vi "Controller_version1.vi"() -> ()   [LabVIEW 2020]
uses:
  <vilib>/Platform/TimedLoop/XDataNode/wakeup.ctl
  <vilib>/Platform/TimedLoop/XDataNode/XDNodeRunTimeDep.lvlib
  <vilib>/Platform/TimedLoop/XDataNode/nitl_modes.ctl
  <vilib>/Platform/TimedLoop/XDataNode/timing_clust.ctl
  <vilib>/Platform/TimedLoop/XDataNode/XDataNode.xnode
  <vilib>/addons/control/pid/NI_PID_pid.lvlib
  <vilib>/addons/control/pid/pid.llb/PID (DBL).vi
  <vilib>/imathl/engines/lvmath/Functions/Error Handling/Create Error.vi
  <vilib>/imath/engines/lvmath2/RunTimeEngine/BuiltInFunctions/diag/NIMS_diag.vi
  <vilib>/imath/engines/lvmath2/RunTimeEngine/NodeEndStatement/NIMS_NodeEndStatement_Output.vi
  <vilib>/imath/engines/lvmath2/RunTimeEngine/ErrorHandling/NIMS_Finalize Error.vi
  <vilib>/imath/engines/lvmath2/RunTimeEngine/IndexReplace/NIMS M($,S)=V.vi
  <vilib>/imath/engines/lvmath2/RunTimeEngine/IndexRead/NIMS V(S).vi
  <vilib>/imath/engines/lvmath2/RunTimeEngine/ErrorHandling/NIMS_Create Error From Enums.vi
  <vilib>/imath/engines/lvmath2/RunTimeEngine/RangeToken/NIMS_Range_R2 - Integer.vi
  <vilib>/imath/engines/lvmath2/RunTimeEngine/VariableToken/NIMS_VariableToken_CondDefinedDefinedByReplace.vi
  <vilib>/imath/engines/lvmath2/RunTimeEngine/IndexReplace/NIMS V(S)=S.vi
  <vilib>/imath/engines/lvmath2/RunTimeEngine/CommandStatement/MC_CommandStatement_break.vi
  <vilib>/imath/engines/lvmath2/RunTimeEngine/VariableToken/NIMS_VariableToken_CondDefined.vi
  <vilib>/imath/engines/lvmath2/RunTimeEngine/IndexRead/NIMS V($).vi
  <vilib>/imath/engines/lvmath2/RunTimeEngine/ArithmeticOperatorToken/NIMS_ArithmeticOperator_rightdiv(C,C).vi
  <vilib>/imath/engines/lvmath2/RunTimeEngine/ArithmeticOperatorToken/NIMS_ArithmeticOperator_minus.vi
  <vilib>/imath/engines/lvmath2/RunTimeEngine/ArithmeticOperatorToken/NIMS_ArithmeticOperator_times.vi
  <vilib>/imath/engines/lvmath2/RunTimeEngine/ArithmeticOperatorToken/NIMS_ArithmeticOperator_plus.vi
  <vilib>/imath/engines/lvmath2/RunTimeEngine/ArithmeticOperatorToken/NIMS_ArithmeticOperator_multmx(M,CV).vi
  <vilib>/imath/engines/lvmath2/RunTimeEngine/ArithmeticOperatorToken/NIMS_ArithmeticOperator_multmx(M,CV)-internal.vi
  <vilib>/imath/engines/lvmath2/RunTimeEngine/ArithmeticOperatorToken/NIMS_ArithmeticOperator_multmx.vi
  <vilib>/imath/engines/lvmath2/RunTimeEngine/ArithmeticOperatorToken/NIMS_ArithmeticOperator_rightdiv.vi
  <vilib>/imath/engines/lvmath2/RunTimeEngine/MatrixToken/NIMS_MatrixToken_SorCV_M.vi
  <vilib>/imath/engines/lvmath2/RunTimeEngine/IndexRead/NIMS V(R2).vi
  <vilib>/imath/engines/lvmath2/RunTimeEngine/BuiltInFunctions/reshapemx/NIMS_[GM]_reshapemx.vi
  <vilib>/imath/engines/lvmath2/RunTimeEngine/IndexRead/NIMS M(S,$).vi
  <vilib>/imath/engines/lvmath2/RunTimeEngine/ArithmeticOperatorToken/NIMS_ArithmeticOperator_multmx(RV,CV).vi
  <vilib>/imath/engines/lvmath2/RunTimeEngine/IndexReplace/NIMS V(S)=M.vi
  <vilib>/imath/engines/lvmath2/RunTimeEngine/IndexRead/NIMS M(S).vi
  <vilib>/imath/engines/lvmath2/RunTimeEngine/ArithmeticOperatorToken/NIMS_ArithmeticOperator_rightdivmx(C,C).vi
  <vilib>/imath/engines/lvmath2/RunTimeEngine/BuiltInFunctions/max/2 inputs/NIMS_max(CG,CG)-no size check.vi
  <vilib>/imath/engines/lvmath2/RunTimeEngine/BuiltInFunctions/min/2 inputs/NIMS_min(CG,CG)-no size check.vi
  <vilib>/imath/engines/lvmath2/RunTimeEngine/IndexReplace/NIMS M(S)=S.vi
  <vilib>/imath/engines/lvmath2/RunTimeEngine/NodeEndStatement/NIMS_NodeEndStatement_Get Vector.vi
  <vilib>/imath/engines/lvmath2/RunTimeEngine/NodeEndStatement/NIMS_NodeEndStatement_Get Scalar.vi
  <vilib>/imath/engines/lvmath/Functions/Error Handling/MergeErrorsWrapper.vi
panel:
  out "No error 3":bool
  out "No error 2":bool
  in  "Use\nPreset_Theta":bool
  out "Theta_Boom_F_hat_next":T1(graph)
  out "Theta_Boom_Q_hat_next":T1(graph)
  out "Theta_Stick_Q_hat_next":T1(graph)
  out "Theta_Stick_F_hat_next":T1(graph)
  out "e2_e3":dbl[](array[numeric])
  out "e3":dbl[](array[numeric])
  out "e2":dbl[](array[numeric])
  out "F_Boom":cluster{dbl, dbl, dbl, dbl}(graph)
  out "Q_Swing":cluster{dbl, dbl, dbl, dbl}(graph)
  in  "保存路径":path=path "C:/Qmz/data1.bin"
  in  "Save Data":bool
  in  "Stop\nTheta_Update":bool=TRUE
  out "Q_Boom":cluster{dbl, dbl, dbl, dbl}(graph)
  out "F_Stick":cluster{dbl, dbl, dbl, dbl}(graph)
  out "Q_Stick":cluster{dbl, dbl, dbl, dbl}(graph)
  out "F_Swing":cluster{dbl, dbl, dbl, dbl}(graph)
  out "Esti_e2":T2(graph)={"FLda1[0]"=125.504748463915, "FLda1[1]"=53.955555282260676, "FLda1[2]"=-93.06627669799211}
  out "Esti_e1":T2(graph)={"FLda1[0]"=125.504748463915, "FLda1[1]"=53.955555282260676, "FLda1[2]"=-93.06627669799211}
  out "Swing":T3(graph)
  out "Stick":T3(graph)
  out "Boom":T3(graph)
  in  "sw_Y_Q":bool
  in  "w2":dbl[](array[numeric])=[1414.0, 4000.0, 3020.0]
  in  "w1":dbl[](array[numeric])=[0.26, 1.1, 0.07]
  out "Theta_Boom_Q_hat_next":dbl[](array[numeric])
  out "Theta_Boom_F_hat_next":dbl[](array[numeric])
  out "Theta_Swing_Q_hat_next":dbl[](array[numeric])
  out "Theta_Swing_F_hat_next":dbl[](array[numeric])
  out "Theta_Stick_Q_hat_next":dbl[](array[numeric])
  out "Theta_Stick_F_hat_next":dbl[](array[numeric])
  out "ARC_U":dbl[](array[numeric])
  in  "sw_d2hat":bool
  in  "sw_d1hat":bool
  in  "gamma_d2(E-8)":dbl[](array[numeric])=[6.5, 3.1, 5.0]
  in  "gamma_d1":dbl[](array[numeric])=[250.0, 6000.1, 6000.1]
  in  "Theta_s2_init(E-8)":dbl[](array[numeric])=[2.0, 2.3, 2.5, 0.0, 100.0, 10.0, 0.0, -99.0, -200.0]
  in  "Theta_s1_init":dbl[](array[numeric])=[500.0, 66.0, 30.0, 53.0, 57.0, 31.0, -10.0, -73.0, 77.0]
  in  "sw_FLda1":bool=TRUE
  in  "sw_QLda1":bool=TRUE
  in  "STOP/Return to save position":bool=TRUE
  in  "Swing？(F)":bool=TRUE
  in  "Boom？(F)":bool
  in  "Stickj？(F)":bool=TRUE
  in  "K3(E-8)":dbl[](array[numeric])=[0.8, 1.0, 4.0] format="%#_8g"
  in  "K2":dbl[](array[numeric])=[650.0, 850.0, 800.0]
  in  "K1":dbl[](array[numeric])=[80.0, 80.0, 80.0]
  out "?":string="Now OpenLoop is running"
  out "?":string="Now OpenLoop is running"
  out "?":string="Now OpenLoop is running"
  in  "CloseLoop":T4 caption="ARC开关"
  out "Angle_Stick":dbl
  out "Angle_Boom":dbl
  out "Angle_Swing":dbl
  out "millisecond timer value":u32
  out "real time(s)":dbl
  out "minus":dbl format="%#_10g"
  out "No error":bool
  in  "PID gains":T5={"proportional gain (Kc)"=0.15, "integral time (Ti, min)"=0.003, "derivative time (Td, min)"=0.0005} caption="未越界" {"derivative time (Td, min)" format="%.6f"; "integral time (Ti, min)" format="%.6f"; "proportional gain (Kc)" step=0.01 format="%.6f"}
  out "?":bool
  in  "PID gains 2":T5={"proportional gain (Kc)"=0.16, "integral time (Ti, min)"=0.006, "derivative time (Td, min)"=0.0001} caption="未越界" {"derivative time (Td, min)" format="%.6f"; "integral time (Ti, min)" format="%.6f"; "proportional gain (Kc)" format="%.6f"}
  in  "PID gains 3":T5={"proportional gain (Kc)"=0.15, "integral time (Ti, min)"=0.003, "derivative time (Td, min)"=1e-05} caption="未越界" {"derivative time (Td, min)" step=0.001 format="%.6f"; "integral time (Ti, min)" step=0.001 format="%.6f"; "proportional gain (Kc)" step=0.01 format="%.6f"}
  out "?":bool
  out "?":bool
  in  "OpenLoop":T6={"Swing"=TRUE, "Boom"=TRUE, "Stick"=TRUE, "Swing_U"=-1.0, "Boom_U"=1.0, "Stick_U"=-1.0}
  in  "bias Swing":dbl
  in  "bias Boom":dbl
  in  "bias Stick":dbl
  in  "t-whole_Swing":i32=300
  in  "p_end Swing":dbl=-40.0
  in  "a_max Swing":dbl=-20.0
  in  "v_max Swing":dbl=-20.0
  in  "t-whole_Boom":i32=300
  in  "p_end Boom":dbl=-40.0
  in  "a_max Boom":dbl=-20.0
  in  "v_max Boom":dbl=-20.0
  in  "t-whole_Stick":i32=300
  in  "p_end_Stick":dbl=-40.0
  in  "a_max_Stick":dbl=-20.0
  in  "v_max_Stick":dbl=-20.0
  in  "pin1":dbl(slide)=40.50458715596331 scale=-60.0..55.0
  in  "Stick":T7={"Open P2P Traj"=TRUE, "Open Sine Traj"=FALSE, "Open Ramp Traj"=FALSE, "Open DIY Traj"=FALSE}
  in  "Boom":T7={"Open P2P Traj"=TRUE, "Open Sine Traj"=FALSE, "Open Ramp Traj"=FALSE, "Open DIY Traj"=FALSE}
  in  "Swing":T7={"Open P2P Traj"=TRUE, "Open Sine Traj"=FALSE, "Open Ramp Traj"=FALSE, "Open DIY Traj"=FALSE}
  in  "pin2":dbl(slide)=33.853211009174316 scale=-20.0..90.0
  in  "pin3":dbl(slide)=-87.9816513761468 scale=-160.0..-53.0
  # "s1 上到下\nfv\nfc\nD_n\ns2 上到下\n1/beta\nD_Q1\nD_Q2"
  # "上到下\n*Ld \\ *Lda1 \\ *Lds2 \\ *Lda2"
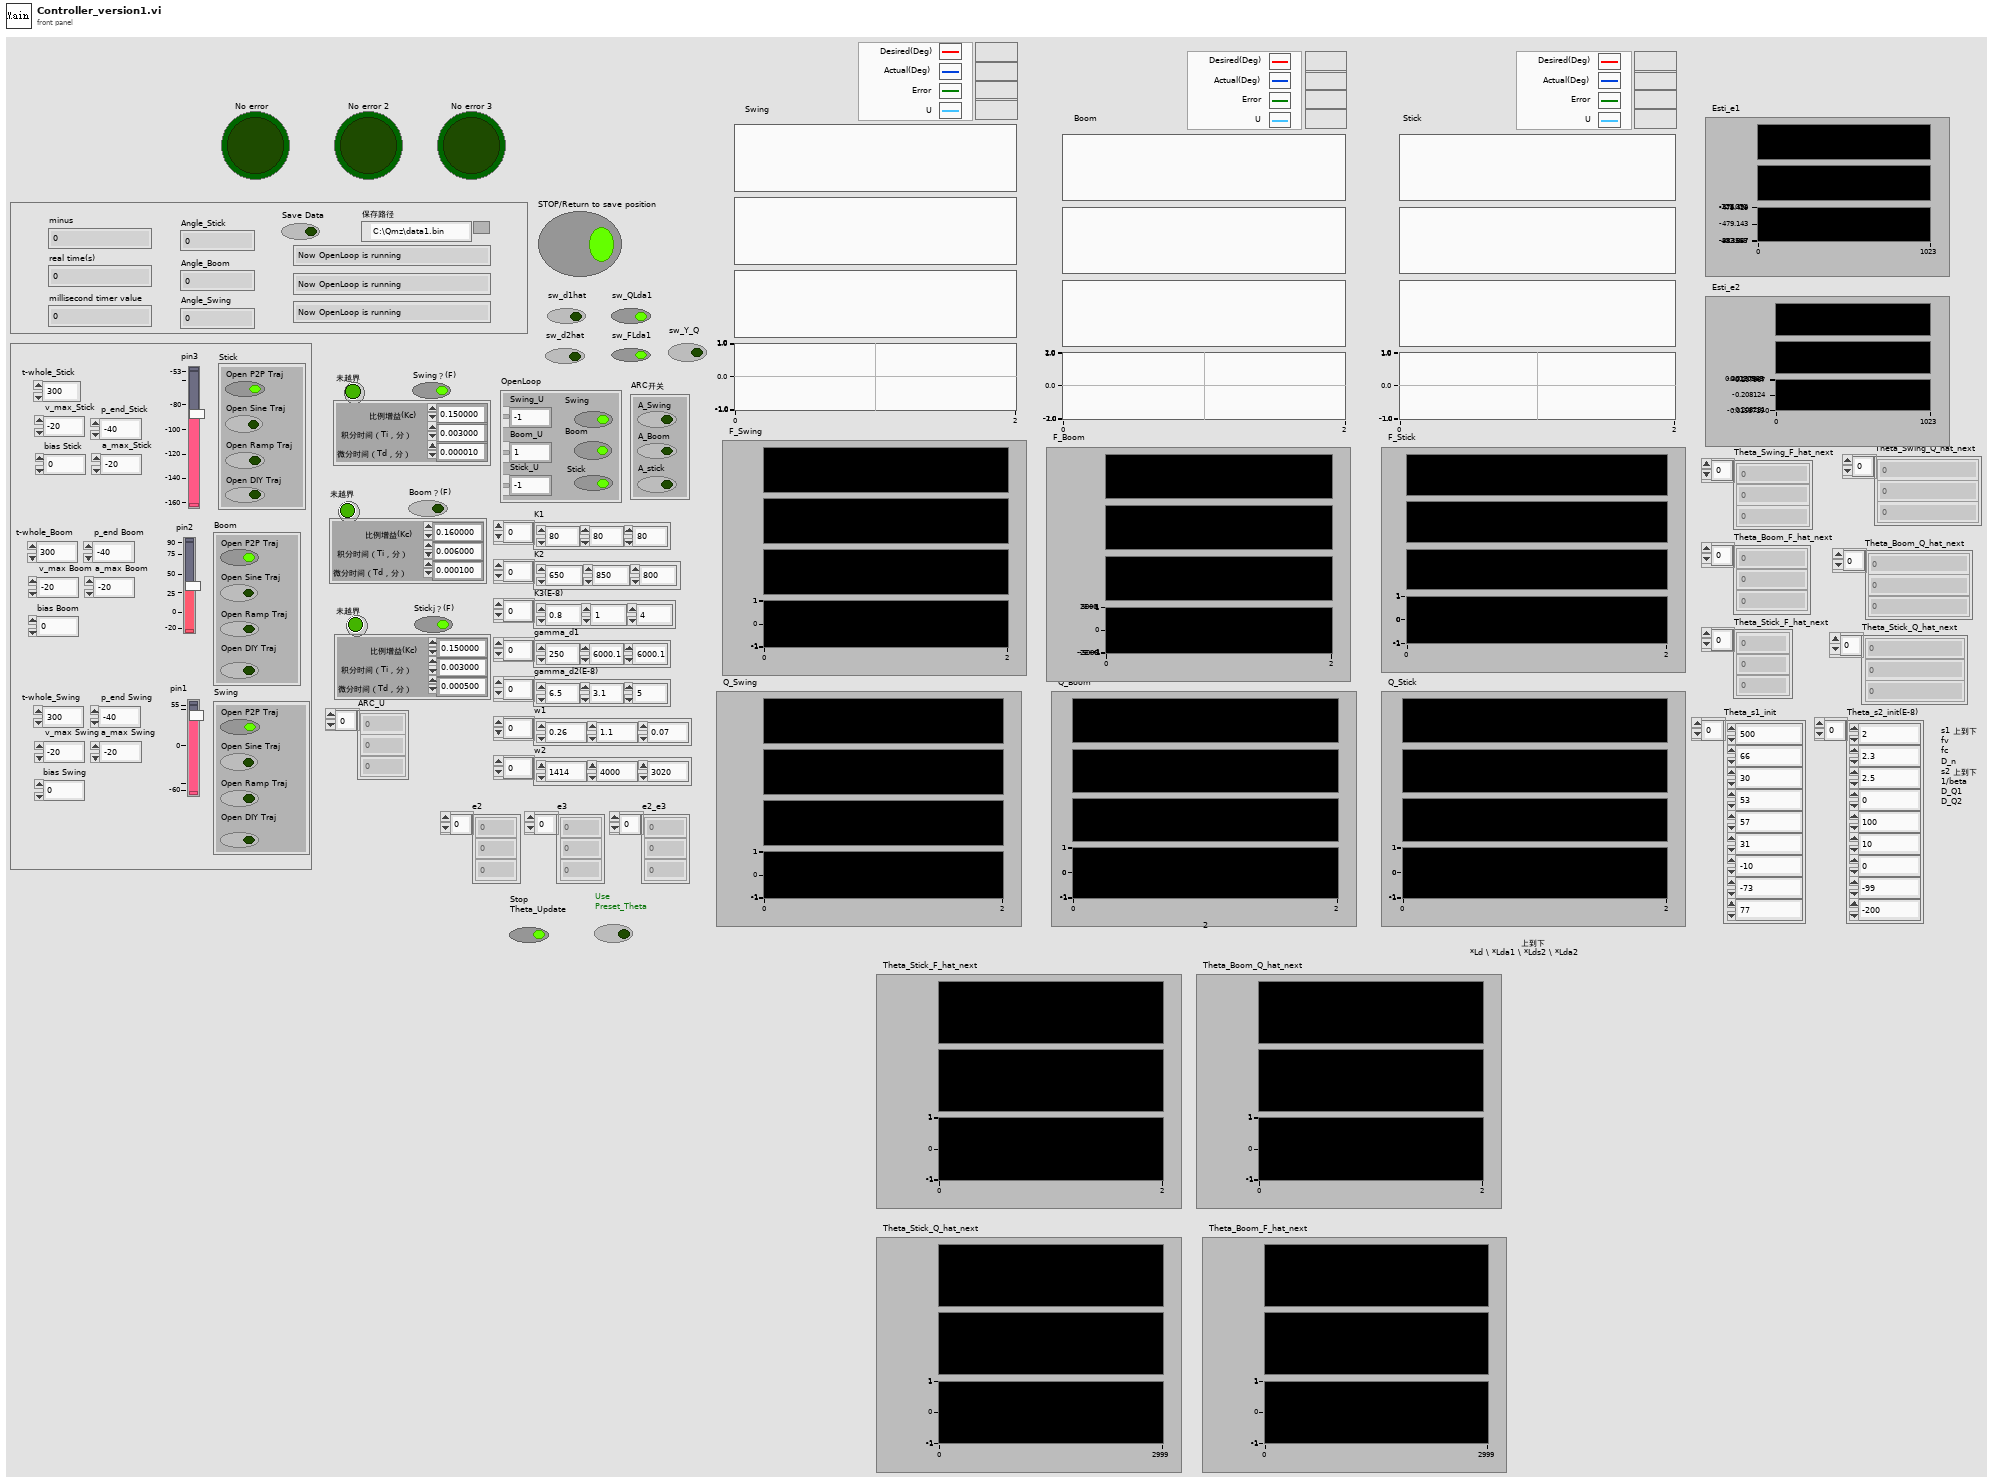
[diagram p1: front panel]
types:
  T1 = cluster{"Theta_Stick_F_hat_next[0]":dbl, "Theta_Stick_F_hat_next[1]":dbl, "Theta_Stick_F_hat_next[2]":dbl}
  T2 = cluster{"FLda1[0]":dbl, "FLda1[1]":dbl, "FLda1[2]":dbl}
  T3 = cluster{"Double":dbl, "Double":dbl, "Double":dbl, "Double":dbl}
  T4 = cluster{"A_Swing":bool, "A_Boom":bool, "A_stick\n":bool}
  T5 = cluster{"proportional gain (Kc)":dbl, "integral time (Ti, min)":dbl, "derivative time (Td, min)":dbl}
  T6 = cluster{"Swing":bool, "Boom":bool, "Stick":bool, "Swing_U":dbl, "Boom_U":dbl, "Stick_U":dbl}
  T7 = cluster{"Open P2P Traj":bool, "Open Sine Traj":bool, "Open Ramp Traj":bool, "Open DIY Traj":bool}
  T8 = typedef "XDNodeRunTimeDep.lvlib/timing_clust.ctl" = cluster{"Expected End [f-1]":u64, "Actual End [f-1]":u64, "Finished Late? [f-1]":bool, "Expected End [i-1]":u64, "Actual End [i-1]":u64, "Finished Late? [i-1]":bool, "Expected Start [i]":u64, "Actual Start [i]":u64, "Expected Start [f]":u64, "Actual Start [f]":u64, "Source Name":string, "Structure Name":string, "Period":i64, "Deadline":i64, "Offset":i64, "Start":i64, "Priority":i32, "Timeout":i32, "Mode":T9, "Wakeup Reason":T10, "Error":errorcluster, "Source Type":string, "Secondary Source Type":string, "Global End Time":u64, "Global Start Time":u64, "Frame Duration":u64, "Iteration Duration":u64, "Assigned CPU":i32, "I/O Scan Engine Mode":u32}
  T9 = typedef "XDNodeRunTimeDep.lvlib/nitl_modes.ctl" = enum32{"No Change", "Process missed periods, maintain original phase", "Discard missed periods, maintain original phase", "Process missed periods, ignore original phase", "Discard missed periods, ignore original phase"}
  T10 = typedef "XDNodeRunTimeDep.lvlib/wakeup.ctl" = enum32{"Normal", "Aborted", "Asynchronous wakeup", "Timing source error", "Timed loop error", "Timeout"}
  T11 = cluster{"Q_Stick[0]":cdb, "Q_Stick[1]":cdb, "Q_Stick[2]":cdb, "Q_Stick[3]":cdb}
  T12 = cluster{"Q_Boom[0]":cdb, "Q_Boom[1]":cdb, "Q_Boom[2]":cdb, "Q_Boom[3]":cdb}
  T13 = cluster{"Q_Swing[0]":cdb, "Q_Swing[1]":cdb, "Q_Swing[2]":cdb, "Q_Swing[3]":cdb}
  T14 = cluster{"F_Stick[0]":cdb, "F_Stick[1]":cdb, "F_Stick[2]":cdb, "F_Stick[3]":cdb}
  T15 = cluster{"F_Boom[0]":cdb, "F_Boom[1]":cdb, "F_Boom[2]":cdb, "F_Boom[3]":cdb}
  T16 = cluster{"F_Swing[0]":cdb, "F_Swing[1]":cdb, "F_Swing[2]":cdb, "F_Swing[3]":cdb}
  T17 = cluster{"Epsilon_1[0]":cdb, "Epsilon_1[1]":cdb, "Epsilon_1[2]":cdb}
  T18 = cluster{"Epsilon_2[0]":cdb, "Epsilon_2[1]":cdb, "Epsilon_2[2]":cdb}
  T19 = cluster{"Theta_Stick_Q_hat_next[0]":dbl, "Theta_Stick_Q_hat_next[1]":dbl, "Theta_Stick_Q_hat_next[2]":dbl}
  T20 = cluster{"Theta_Boom_Q_hat_next[0]":dbl, "Theta_Boom_Q_hat_next[1]":dbl, "Theta_Boom_Q_hat_next[2]":dbl}
  T21 = cluster{"Theta_Boom_F_hat_next[0]":dbl, "Theta_Boom_F_hat_next[1]":dbl, "Theta_Boom_F_hat_next[2]":dbl}
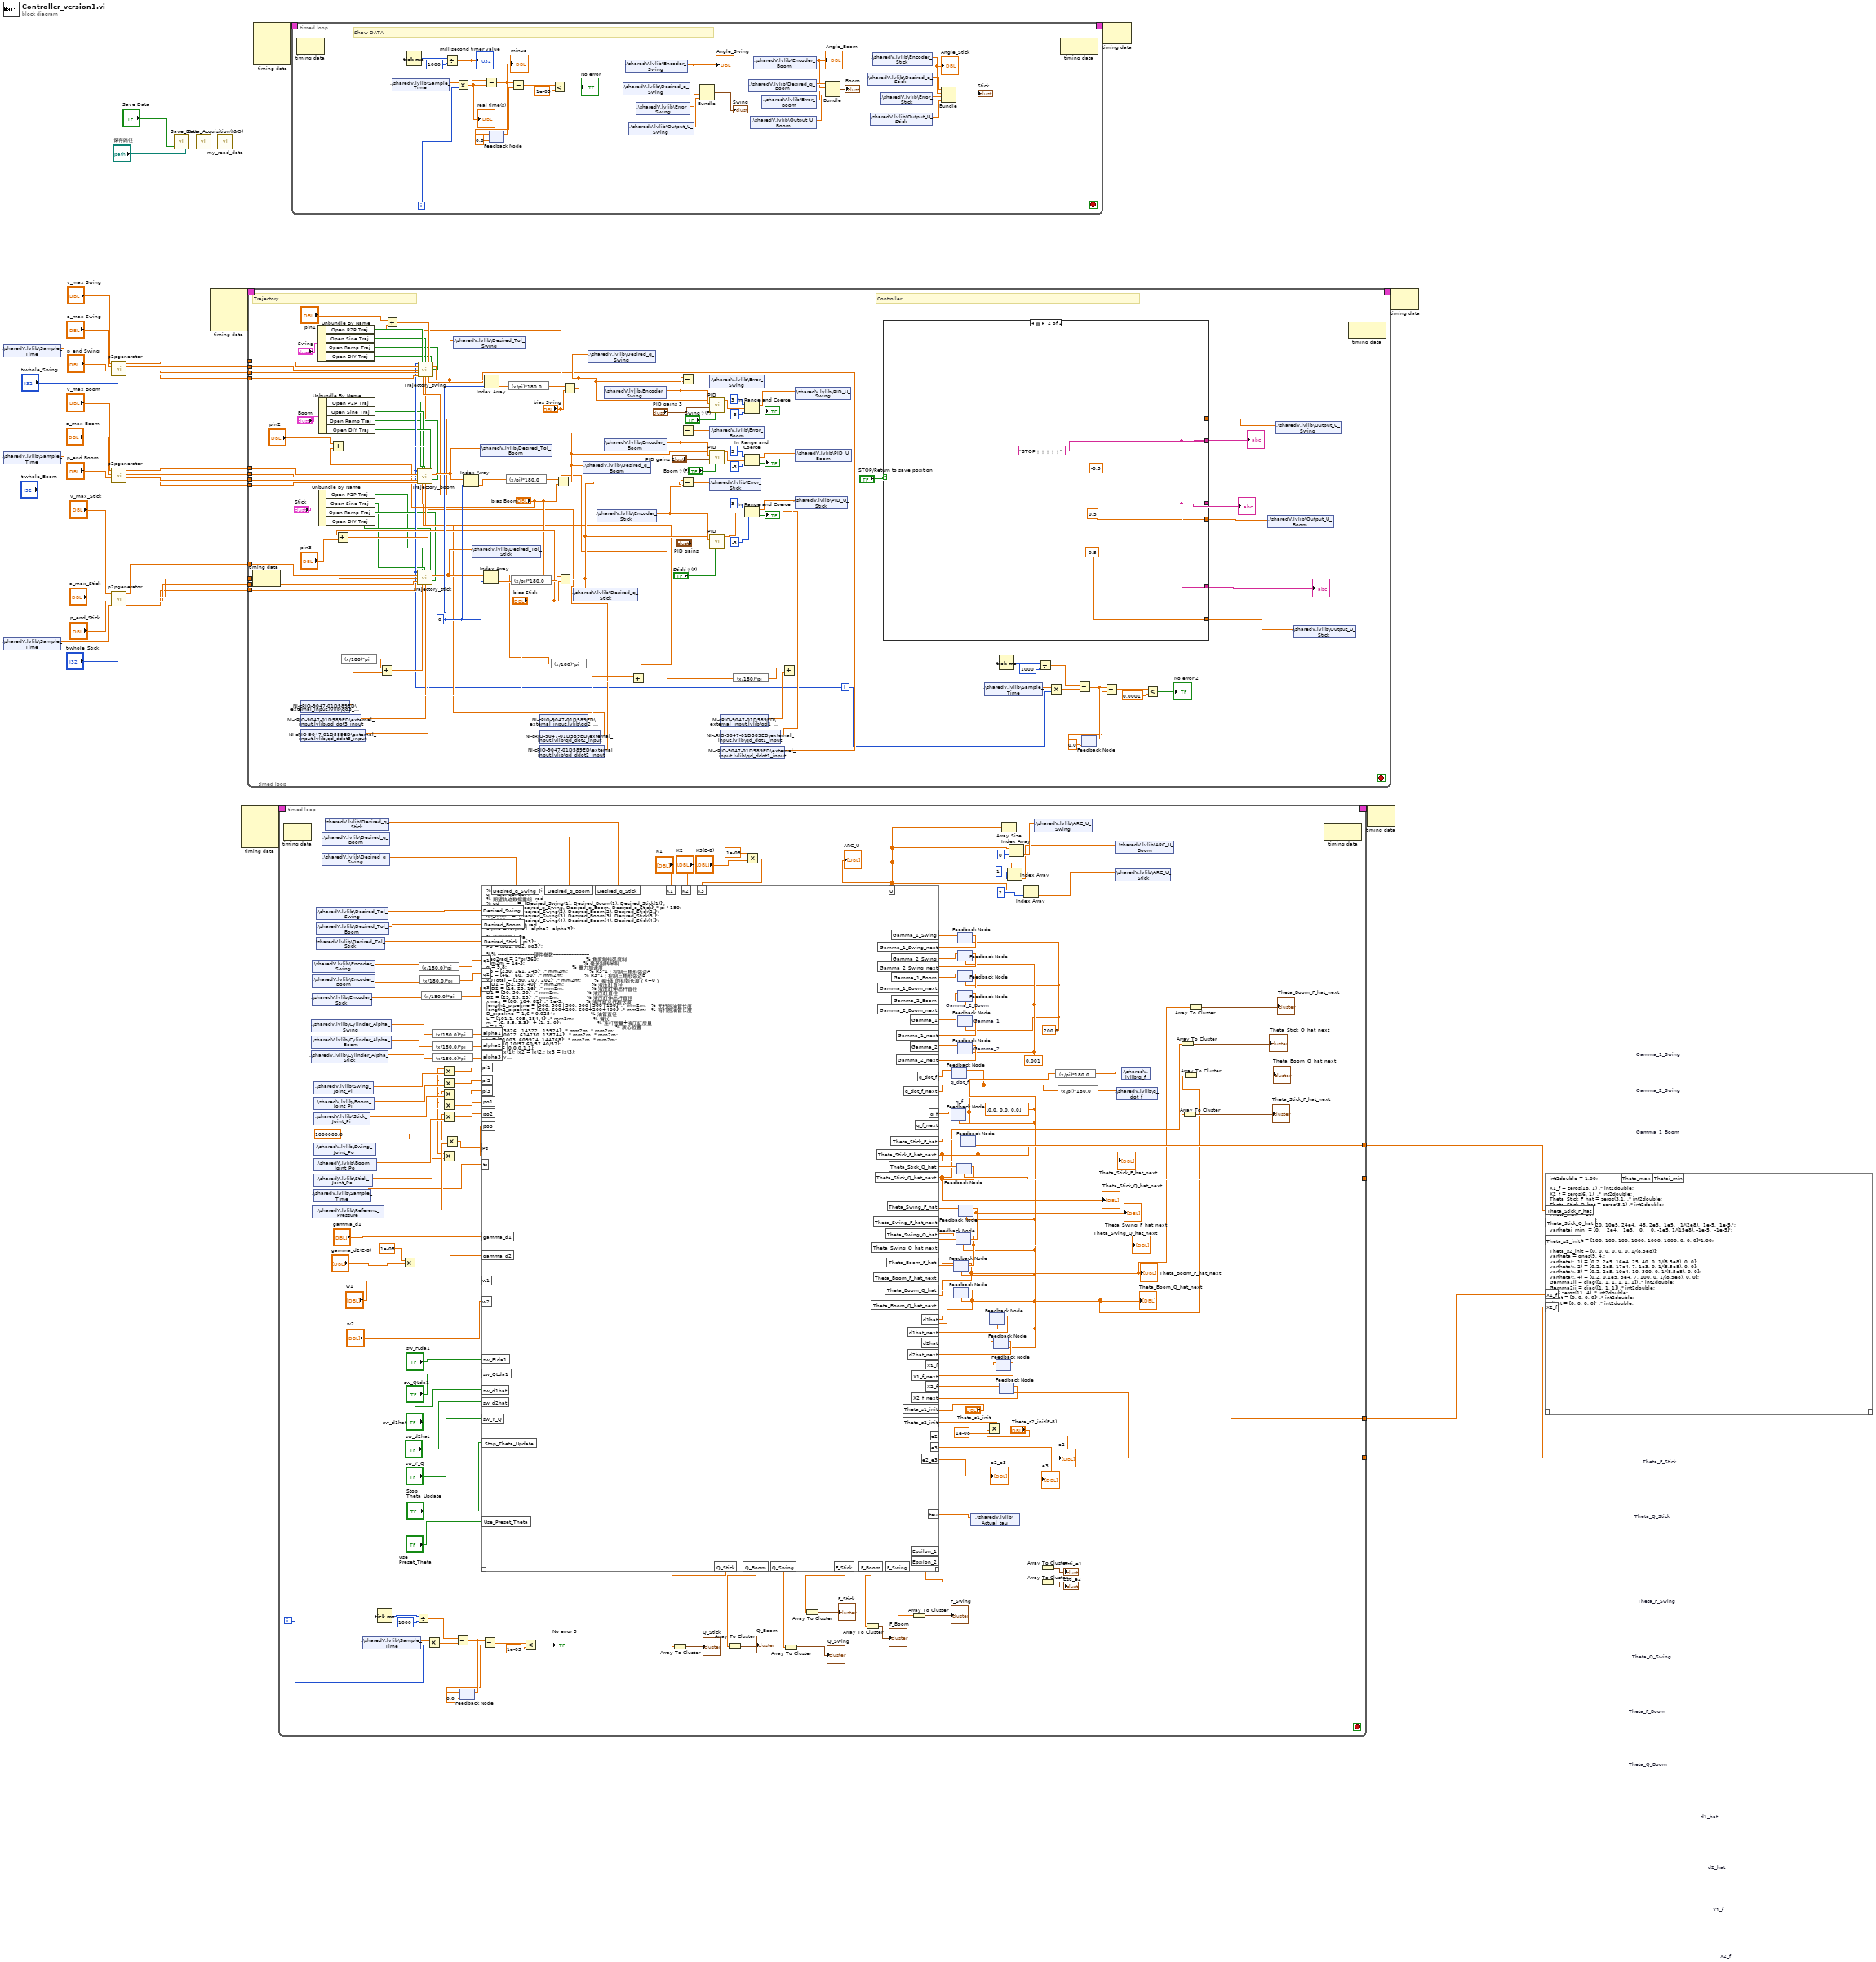
[diagram p0: block diagram]
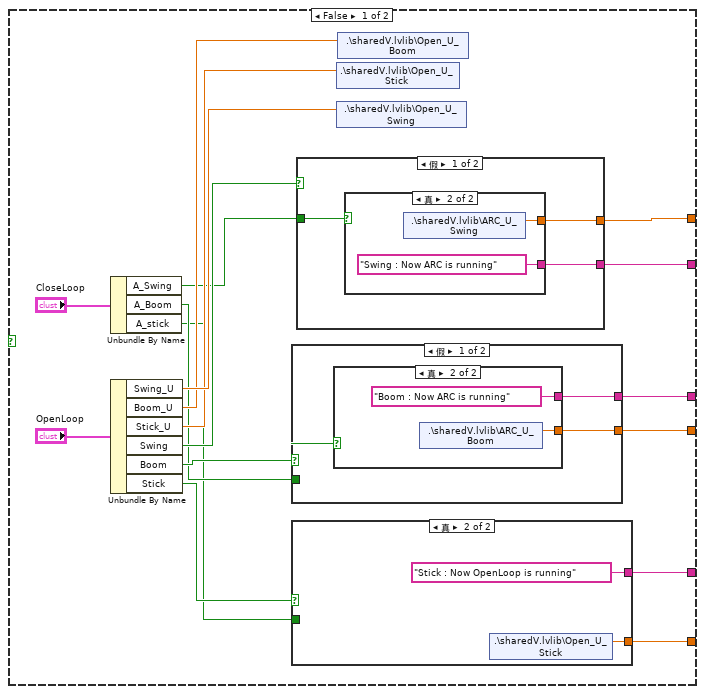
[diagram p2: hidden frame]
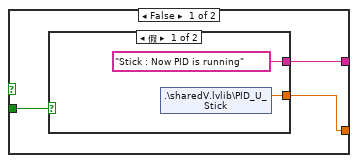
[diagram p3: hidden frame]
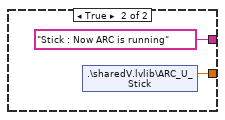
[diagram p4: hidden frame]
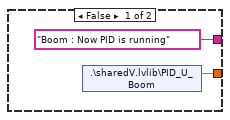
[diagram p5: hidden frame]
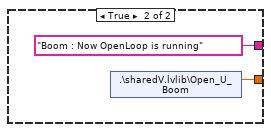
[diagram p6: hidden frame]
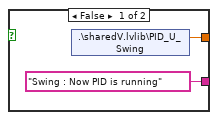
[diagram p7: hidden frame]
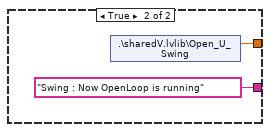
[diagram p8: hidden frame]
diagram:
  n1 = shared-variable ".\\sharedV.lvlib\\Sample_Time"() -> (w20:dbl)  [unwired: 1 in, 1 out]
  n2 = shared-variable ".\\sharedV.lvlib\\Sample_Time"() -> (w25:dbl)  [unwired: 1 in, 1 out]
  n3 = shared-variable ".\\sharedV.lvlib\\Sample_Time"() -> (w3:dbl)  [unwired: 1 in, 1 out]
  n4 = call "p2pgenerator.vi"("whole time for p2p"="t-whole_Swing", "ts"=w20, "p_end"="p_end Swing", "a_max"="a_max Swing", "v_max"="v_max Swing") -> ("jerk"=w12:dbl[], "a"=w13:dbl[], "v"=w14:dbl[], "s"=w15:dbl[])  [unwired: 3 in]
  n5 = call "p2pgenerator.vi"("whole time for p2p"="t-whole_Boom", "ts"=w25, "p_end"="p_end Boom", "a_max"="a_max Boom", "v_max"="v_max Boom") -> ("jerk"=w16:dbl[], "a"=w17:dbl[], "v"=w18:dbl[], "s"=w19:dbl[])  [unwired: 3 in]
  n6 = call "p2pgenerator.vi"("whole time for p2p"="t-whole_Stick", "ts"=w3, "p_end"="p_end_Stick", "a_max"="a_max_Stick", "v_max"="v_max_Stick") -> ("jerk"=w30:dbl[], "a"=w31:dbl[], "v"=w32:dbl[], "s"=w33:dbl[])  [unwired: 3 in]
  n7 = call "Save_Data.vi"("保存路径"="保存路径", "Save Data"="Save Data") -> ()  [unwired: 4 in]
  n8 = call "Data_Acquisition(I&O).vi"() -> ()  [unwired: 12 in]
  n9 = node-c288() -> (w39:T8)  [unwired: 4 in]
  n10 = call "my_read_data.vi"() -> ()  [unwired: 12 in]
  n11 = node-c288() -> (w9:T8)  [unwired: 4 in]
  n12 = timed-loop "定时循环" {
    timing: w39 -> [_]
    timing-out: [_] -> w38
    tunnel: w33 -> [w146]
    tunnel: w32 -> [w149]
    tunnel: w31 -> [w148]
    tunnel: w30 -> [w147]
    tunnel: w19 -> [w145]
    tunnel: w18 -> [w144]
    tunnel: w17 -> [w143]
    tunnel: w16 -> [w142]
    tunnel: w15 -> [w136]
    tunnel: w14 -> [w135]
    tunnel: w13 -> [w134]
    tunnel: w12 -> [w133]
    i -> [w50]
    stop <- _ stop-if-true
    w107 = 0
    # "Controller"
    # "Trajectory"
    n13 = node-c288() -> ()  [unwired: 1 in, 1 out]
    n14 = shared-variable "NI-cRIO-9047-01D589ED\\external_input.lvlib\\qd3_input"() -> (w75:dbl[])  [unwired: 1 in, 1 out]
    n15 = shared-variable "NI-cRIO-9047-01D589ED\\external_input.lvlib\\qd_dot3_input"() -> (w76:dbl[])  [unwired: 1 in, 1 out]
    n16 = shared-variable "NI-cRIO-9047-01D589ED\\external_input.lvlib\\qd_ddot3_input"() -> (w77:dbl[])  [unwired: 1 in, 1 out]
    n17 = Unbundle By Name ("按名称解除捆绑")("Swing") -> ("Open P2P Traj"=w138:bool, "Open Sine Traj"=w137:bool, "Open Ramp Traj"=w41:bool, "Open DIY Traj"=w40:bool)
    n18 = Unbundle By Name ("按名称解除捆绑")("Stick") -> ("Open P2P Traj"=w46:bool, "Open Sine Traj"=w47:bool, "Open Ramp Traj"=w48:bool, "Open DIY Traj"=w49:bool)
    n19 = Unbundle By Name ("按名称解除捆绑")("Boom") -> ("Open P2P Traj"=w43:bool, "Open Sine Traj"=w44:bool, "Open Ramp Traj"=w42:bool, "Open DIY Traj"=w45:bool)
    n20 = Add ("加")(x="pin2", y="bias Boom") -> (x+y=w83:dbl)
    n21 = Add ("加")(x="bias Stick", y="pin3") -> (x+y=w84:dbl)
    n22 = expression code="(x/180)*pi" ("弧度转换至角度")("bias Stick") -> (w78:dbl)
    n23 = Add ("加")(x=w78, y=w75) -> (x+y=w74:dbl[])
    n24 = Add ("加")(x="pin1", y="bias Swing") -> (x+y=w80:dbl)
    n25 = call "Trajectory_stick.vi"("i"=w50, "if p2p"=w46, "ifSin?"=w47, "Target_Angle"=w84, "if_DIY"=w49, "q"=w146, "qd"=w149, "qdd"=w148, "if_Ramp"=w48, "qddd"=w147, "qd8_1"=w74, "qd8_dot_2"=w76, "qd8_ddot_2"=w77) -> ("qd1_tol"=w86:dbl[])  [unwired: 2 in]
    n26 = shared-variable ".\\sharedV.lvlib\\Desired_Tol_Stick"(w86) -> ()  [unwired: 1 in, 1 out]
    n27 = Index Array ("索引数组")(array=w86, index=w107) -> (element=w104:dbl)
    n28 = expression code="(x/pi)*180.0" ("弧度转换至角度")(w104) -> (w103:dbl)
    n29 = shared-variable "NI-cRIO-9047-01D589ED\\external_input.lvlib\\qd2_input"() -> (w73:dbl[])  [unwired: 1 in, 1 out]
    n30 = shared-variable "NI-cRIO-9047-01D589ED\\external_input.lvlib\\qd_dot2_input"() -> (w69:dbl[])  [unwired: 1 in, 1 out]
    n31 = shared-variable "NI-cRIO-9047-01D589ED\\external_input.lvlib\\qd_ddot2_input"() -> (w68:dbl[])  [unwired: 1 in, 1 out]
    n32 = expression code="(x/180)*pi" ("弧度转换至角度")("bias Boom") -> (w71:dbl)
    n33 = Subtract ("减")(x=w103, y="bias Stick") -> (x-y=w97:dbl)
    n34 = shared-variable ".\\sharedV.lvlib\\Desired_q_Stick"(w97) -> ()  [unwired: 1 in, 1 out]
    n35 = shared-variable ".\\sharedV.lvlib\\Encoder_Stick"() -> (w98:dbl)  [unwired: 1 in, 1 out]
    n36 = shared-variable ".\\sharedV.lvlib\\Encoder_Swing"() -> (w94:dbl)  [unwired: 1 in, 1 out]
    n37 = shared-variable ".\\sharedV.lvlib\\Encoder_Boom"() -> (w96:dbl)  [unwired: 1 in, 1 out]
    n38 = Add ("加")(x=w73, y=w71) -> (x+y=w70:dbl[])
    n39 = call "Trajectory_boom.vi"("i"=w50, "if p2p"=w43, "ifSin?"=w44, "Target_Angle"=w83, "if end8"=w45, "q"=w145, "qd"=w144, "qdd"=w143, "if  Ramp"=w42, "qddd"=w142, "qd8_1"=w70, "qd8_dot_2"=w69, "qd8_ddot_2"=w68) -> ("qd1_tol"=w111:dbl[])  [unwired: 2 in]
    n40 = Index Array ("索引数组")(array=w111, index=w107) -> (element=w110:dbl)
    n41 = shared-variable ".\\sharedV.lvlib\\Desired_Tol_Boom"(w111) -> ()  [unwired: 1 in, 1 out]
    n42 = expression code="(x/pi)*180.0" ("弧度转换至角度")(w110) -> (w132:dbl)
    n43 = Subtract ("减")(x=w132, y="bias Boom") -> (x-y=w95:dbl)
    n44 = shared-variable ".\\sharedV.lvlib\\Desired_q_Boom"(w95) -> ()  [unwired: 1 in, 1 out]
    n45 = Subtract ("减")(x=w96, y=w95) -> (x-y=w109:dbl)
    n46 = Subtract ("减")(x=w98, y=w97) -> (x-y=w91:dbl)
    n47 = shared-variable ".\\sharedV.lvlib\\Error_Boom"(w109) -> ()  [unwired: 1 in, 1 out]
    n48 = call-poly <vilib>:"PID.vi"("reinitialize? (F)"="Boom？(F)", "PID gains"="PID gains 2", "process variable"=w96, "setpoint"=w95) -> ("output"=w125:dbl)  [unwired: 6 in, 1 out]
    n49 = shared-variable ".\\sharedV.lvlib\\Error_Stick"(w91) -> ()  [unwired: 1 in, 1 out]
    n50 = call-poly <vilib>:"PID.vi"("reinitialize? (F)"="Stickj？(F)", "PID gains"="PID gains", "process variable"=w98, "setpoint"=w97) -> ("output"=w102:dbl)  [unwired: 6 in, 1 out]
    n51 = shared-variable "NI-cRIO-9047-01D589ED\\external_input.lvlib\\qd1_input"() -> (w65:dbl[])  [unwired: 1 in, 1 out]
    n52 = shared-variable "NI-cRIO-9047-01D589ED\\external_input.lvlib\\qd_dot1_input"() -> (w63:dbl[])  [unwired: 1 in, 1 out]
    n53 = shared-variable "NI-cRIO-9047-01D589ED\\external_input.lvlib\\qd_ddot1_input"() -> (w62:dbl[])  [unwired: 1 in, 1 out]
    n54 = expression code="(x/180)*pi" ("弧度转换至角度")("bias Swing") -> (w66:dbl)
    n55 = In Range and Coerce ("判定范围并强制转换")(upper limit=3, x=w125, lower limit=-3) -> (coerced(x)=w116:dbl, In Range?=→"?":bool)
    n56 = In Range and Coerce ("判定范围并强制转换")(upper limit=3, x=w102, lower limit=-3) -> (coerced(x)=w117:dbl, In Range?=→"?":bool)
    n57 = Add ("加")(x=w66, y=w65) -> (x+y=w64:dbl[])
    n58 = call "Trajectory_swing.vi"("i"=w50, "if p2p"=w138, "ifSin?"=w137, "Target_Angle"=w80, "if end8"=w40, "q"=w136, "qd"=w135, "if Ramp"=w41, "qdd"=w134, "qddd"=w133, "qd8_1"=w64, "qd8_dot_2"=w63, "qd8_ddot_2"=w62) -> ("qd1_tol"=w108:dbl[])  [unwired: 2 in]
    n59 = shared-variable ".\\sharedV.lvlib\\Desired_Tol_Swing"(w108) -> ()  [unwired: 1 in, 1 out]
    n60 = Index Array ("索引数组")(array=w108, index=w107) -> (element=w106:dbl)
    n61 = expression code="(x/pi)*180.0" ("弧度转换至角度")(w106) -> (w87:dbl)
    n62 = Subtract ("减")(x=w87, y="bias Swing") -> (x-y=w93:dbl)
    n63 = shared-variable ".\\sharedV.lvlib\\Desired_q_Swing"(w93) -> ()  [unwired: 1 in, 1 out]
    n64 = Subtract ("减")(x=w94, y=w93) -> (x-y=w105:dbl)
    n65 = shared-variable ".\\sharedV.lvlib\\Error_Swing"(w105) -> ()  [unwired: 1 in, 1 out]
    n66 = call-poly <vilib>:"PID.vi"("reinitialize? (F)"="Swing？(F)", "PID gains"="PID gains 3", "process variable"=w94, "setpoint"=w93) -> ("output"=w131:dbl)  [unwired: 6 in, 1 out]
    n67 = In Range and Coerce ("判定范围并强制转换")(upper limit=3, x=w131, lower limit=-3) -> (coerced(x)=w115:dbl, In Range?=→"?":bool)
    n68 = shared-variable ".\\sharedV.lvlib\\PID_U_Swing"(w115) -> ()  [unwired: 1 in, 1 out]
    n69 = shared-variable ".\\sharedV.lvlib\\PID_U_Boom"(w116) -> ()  [unwired: 1 in, 1 out]
    n70 = shared-variable ".\\sharedV.lvlib\\PID_U_Stick"(w117) -> ()  [unwired: 1 in, 1 out]
    n71 = case "条件结构" shown="真" "STOP/Return to save position" {
      tunnel: [w160 -0.5] -> w90
      tunnel: [w158 w197] -> w114
      tunnel: [w155 w197] -> w113
      tunnel: [w154 0.5] -> w89
      tunnel: [w153 w197] -> w112
      tunnel: [w152 -0.5] -> w88
      frame False {
        n72 = Unbundle By Name ("按名称解除捆绑")("CloseLoop") -> ("A_Swing"=w159:bool, "A_Boom"=w156:bool, "A_stick"=w150:bool)
        n73 = Unbundle By Name ("按名称解除捆绑")("OpenLoop") -> ("Swing_U"=w165:dbl, "Boom_U"=w163:dbl, "Stick_U"=w162:dbl, "Swing"=w161:bool, "Boom"=w157:bool, "Stick"=w151:bool)
        n74 = case "条件结构" shown="假" w157 {
          tunnel: [w176 w184] -> w154
          tunnel: w156 -> [w178 _]
          tunnel: [w177 "Boom : Now OpenLoop is running"] -> w155
          frame False {
            n75 = case "条件结构" shown="真" w178 {
              tunnel: ["Boom : Now PID is running" "Boom : Now ARC is running"] -> w177
              tunnel: [w179 w181] -> w176
              frame False {
                n76 = shared-variable ".\\sharedV.lvlib\\PID_U_Boom"() -> (w179:dbl)  [unwired: 1 in, 1 out]
              }
              frame True {
                n77 = shared-variable ".\\sharedV.lvlib\\ARC_U_Boom"() -> (w181:dbl)  [unwired: 1 in, 1 out]
              }
            }
          }
          frame True {
            n78 = shared-variable ".\\sharedV.lvlib\\Open_U_Boom"() -> (w184:dbl)  [unwired: 1 in, 1 out]
          }
        }
        n79 = case "条件结构" shown="真" w151 {
          tunnel: [w167 w175] -> w152
          tunnel: w150 -> [w169 _]
          tunnel: [w168 "Stick : Now OpenLoop is running"] -> w153
          frame False {
            n80 = case "条件结构" shown="假" w169 {
              tunnel: ["Stick : Now PID is running" "Stick : Now ARC is running"] -> w168
              tunnel: [w170 w172] -> w167
              frame False {
                n81 = shared-variable ".\\sharedV.lvlib\\PID_U_Stick"() -> (w170:dbl)  [unwired: 1 in, 1 out]
              }
              frame True {
                n82 = shared-variable ".\\sharedV.lvlib\\ARC_U_Stick"() -> (w172:dbl)  [unwired: 1 in, 1 out]
              }
            }
          }
          frame True {
            n83 = shared-variable ".\\sharedV.lvlib\\Open_U_Stick"() -> (w175:dbl)  [unwired: 1 in, 1 out]
          }
        }
        n84 = case "条件结构" shown="假" w161 {
          tunnel: [w185 w193] -> w160
          tunnel: w159 -> [w187 _]
          tunnel: [w186 "Swing : Now OpenLoop is running"] -> w158
          frame False {
            n85 = case "条件结构" shown="真" w187 {
              tunnel: ["Swing : Now PID is running" "Swing : Now ARC is running"] -> w186
              tunnel: [w188 w190] -> w185
              frame False {
                n86 = shared-variable ".\\sharedV.lvlib\\PID_U_Swing"() -> (w188:dbl)  [unwired: 1 in, 1 out]
              }
              frame True {
                n87 = shared-variable ".\\sharedV.lvlib\\ARC_U_Swing"() -> (w190:dbl)  [unwired: 1 in, 1 out]
              }
            }
          }
          frame True {
            n88 = shared-variable ".\\sharedV.lvlib\\Open_U_Swing"() -> (w193:dbl)  [unwired: 1 in, 1 out]
          }
        }
        n89 = shared-variable ".\\sharedV.lvlib\\Open_U_Stick"(w162) -> ()  [unwired: 1 in, 1 out]
        n90 = shared-variable ".\\sharedV.lvlib\\Open_U_Swing"(w165) -> ()  [unwired: 1 in, 1 out]
        n91 = shared-variable ".\\sharedV.lvlib\\Open_U_Boom"(w163) -> ()  [unwired: 1 in, 1 out]
      }
      frame True {
        w197 = "STOP！！！！！"
      }
    }
    "?" <- w114
    "?" <- w113
    "?" <- w112
    n92 = shared-variable ".\\sharedV.lvlib\\Sample_Time"() -> (w61:dbl)  [unwired: 1 in, 1 out]
    n93 = Tick Count (ms) ("时间计数器")() -> (millisecond timer value=w59:u32)
    n94 = Divide ("除")(x=w59, y=u32 1000) -> (x/y=w57:dbl)
    n95 = Multiply ("乘")(x=w61, y=w50) -> (x*y=w60:dbl)
    n96 = Subtract ("减")(x=w57, y=w60) -> (x-y=w53:dbl)
    n97 = feedback #1 ("反馈节点")(0.0) -> (w52:dbl)
    n98 = feedback-in #1(w53) -> ()
    n99 = Subtract ("减")(x=w53, y=w52) -> (x-y=w56:dbl)
    n100 = Less? ("小于？")(x=w56, y=0.0001) -> (x < y?=→"No error 2":bool)
    n101 = shared-variable ".\\sharedV.lvlib\\Output_U_Boom"(w89) -> ()  [unwired: 1 in, 1 out]
    n102 = shared-variable ".\\sharedV.lvlib\\Output_U_Swing"(w90) -> ()  [unwired: 1 in, 1 out]
    n103 = shared-variable ".\\sharedV.lvlib\\Output_U_Stick"(w88) -> ()  [unwired: 1 in, 1 out]
    n104 = node-c288() -> ()  [unwired: 1 in, 1 out]
  }
  n105 = node-c288() -> (w11:T8)  [unwired: 4 in]
  n106 = timed-loop "定时循环" {
    timing: w11 -> [_]
    timing-out: [_] -> w10
    i -> [w215]
    stop <- _ stop-if-true
    # "Show DATA"
    n107 = node-c288() -> ()  [unwired: 1 in, 1 out]
    n108 = shared-variable ".\\sharedV.lvlib\\Sample_Time"() -> (w226:dbl)  [unwired: 1 in, 1 out]
    n109 = Tick Count (ms) ("时间计数器")() -> (millisecond timer value=w224:u32)
    n110 = Divide ("除")(x=w224, y=u32 1000) -> (x/y=w222:dbl)
    "millisecond timer value" <- w222
    n111 = Multiply ("乘")(x=w226, y=w215) -> (x*y=w225:dbl)
    "real time(s)" <- w225
    n112 = Subtract ("减")(x=w222, y=w225) -> (x-y=w218:dbl)
    "minus" <- w218
    n113 = feedback #2 ("反馈节点")(0.0) -> (w217:dbl)
    n114 = feedback-in #2(w218) -> ()
    n115 = Subtract ("减")(x=w218, y=w217) -> (x-y=w221:dbl)
    n116 = Less? ("小于？")(x=w221, y=1e-05) -> (x < y?=→"No error":bool)
    n117 = shared-variable ".\\sharedV.lvlib\\Desired_q_Swing"() -> (w214:dbl)  [unwired: 1 in, 1 out]
    n118 = shared-variable ".\\sharedV.lvlib\\Encoder_Swing"() -> (w206:dbl)  [unwired: 1 in, 1 out]
    "Angle_Swing" <- w206
    n119 = shared-variable ".\\sharedV.lvlib\\Output_U_Swing"() -> (w212:dbl)  [unwired: 1 in, 1 out]
    n120 = shared-variable ".\\sharedV.lvlib\\Error_Swing"() -> (w213:dbl)  [unwired: 1 in, 1 out]
    n121 = Bundle ("捆绑")("Double"=w214, "Double"=w206, "Double"=w213, "Double"=w212) -> (→"Swing":T3)  [unwired: 1 in]
    n122 = shared-variable ".\\sharedV.lvlib\\Desired_q_Boom"() -> (w210:dbl)  [unwired: 1 in, 1 out]
    n123 = shared-variable ".\\sharedV.lvlib\\Output_U_Boom"() -> (w207:dbl)  [unwired: 1 in, 1 out]
    n124 = shared-variable ".\\sharedV.lvlib\\Encoder_Boom"() -> (w209:dbl)  [unwired: 1 in, 1 out]
    "Angle_Boom" <- w209
    n125 = shared-variable ".\\sharedV.lvlib\\Error_Boom"() -> (w208:dbl)  [unwired: 1 in, 1 out]
    n126 = Bundle ("捆绑")("Double"=w210, "Double"=w209, "Double"=w208, "Double"=w207) -> (→"Boom":T3)  [unwired: 1 in]
    n127 = shared-variable ".\\sharedV.lvlib\\Desired_q_Stick"() -> (w203:dbl)  [unwired: 1 in, 1 out]
    n128 = shared-variable ".\\sharedV.lvlib\\Output_U_Stick"() -> (w205:dbl)  [unwired: 1 in, 1 out]
    n129 = shared-variable ".\\sharedV.lvlib\\Encoder_Stick"() -> (w202:dbl)  [unwired: 1 in, 1 out]
    "Angle_Stick" <- w202
    n130 = shared-variable ".\\sharedV.lvlib\\Error_Stick"() -> (w204:dbl)  [unwired: 1 in, 1 out]
    n131 = Bundle ("捆绑")("Double"=w203, "Double"=w202, "Double"=w204, "Double"=w205) -> (→"Stick":T3)  [unwired: 1 in]
    n132 = node-c288() -> ()  [unwired: 1 in, 1 out]
  }
  n133 = node-c288(w10) -> ()  [unwired: 1 out]
  n134 = node-c288(w38) -> ()  [unwired: 1 out]
  n135 = mathscript code="int2double = 1.00;\n\nX1_f = zeros(18, 1) .* int2double;\nX2_f = zeros(6, 1)  .* int2double;\nTheta_Stick_F_hat = zeros(3,1) .* int2double;\nTheta_Stick_Q_hat = zeros(3,1) .* int2double;\n\nTheta_max = 20;\nThetai_min  = -20;\nvarthetai_max = [20, 10e5, 24e4,  48, 2e3,  1e5,   1/(2e8),  1e-5,  1e-5]';\nvarthetai_min  = [0,    2e4,   1e3,   0,    0, -1e5, 1/(15e8), -1e-5,  -1e-5]';\n\nTheta_s1_init = [100, 100, 100, 1000, 1000, 1000, 0, 0, 0]*1.00;\n\nTheta_s2_init = [0, 0, 0, 0, 0, 0, 1/(8.5e8)];\nvartheta = ones(9, 4);\nvartheta(:, 1) = [0.2, 2e5, 16e4, 25, 40, 0, 1/(8.5e8), 0, 0];\nvartheta(:, 2) = [0.2, 2e5, 17e4, 7, 1e3, 0, 1/(8.5e8), 0, 0];\nvartheta(:, 3) = [0.2, 2e5, 10e4, 10, 300, 0, 1/(8.5e8), 0, 0];\nvartheta(:, 4) = [0.2, 0.1e5, 5e4, 7, 100, 0, 1/(8.5e8), 0, 0];\nGamma1ii = diag([1, 1, 1, 1, 1, 1]) .* int2double;\nGamma2ii = diag([1, 1, 1]) .* int2double;\nXf = zeros(11, 4) .* int2double;\ndihat = [0, 0, 0, 0]' .* int2double;\nzihat = [0, 0, 0, 0]' .* int2double;"() -> ("Theta_Stick_F_hat"=w5:dbl[], "X1_f"=w7:dbl[], "X2_f"=w6:dbl[], "Theta_Stick_Q_hat"=w4:dbl[])  [unwired: 1 in, 4 out]
  n136 = timed-loop "定时循环" {
    timing: w9 -> [_]
    timing-out: [_] -> w8
    tunnel: w7 -> [w310]
    tunnel: w6 -> [w309]
    tunnel: w5 -> [w307]
    tunnel: w4 -> [w305]
    i -> [w233]
    stop <- _ stop-if-true
    w260 = 0.001
    w259 = 200.0
    w275 = dbl[] [0.0, 0.0, 0.0]
    w350 = 1000000.0
    n137 = node-c288() -> ()  [unwired: 1 in, 1 out]
    n138 = shared-variable ".\\sharedV.lvlib\\Cylinder_Alpha_Swing"() -> (w371:dbl)  [unwired: 1 in, 1 out]
    n139 = shared-variable ".\\sharedV.lvlib\\Cylinder_Alpha_Boom"() -> (w368:dbl)  [unwired: 1 in, 1 out]
    n140 = shared-variable ".\\sharedV.lvlib\\Cylinder_Alpha_Stick"() -> (w367:dbl)  [unwired: 1 in, 1 out]
    n141 = shared-variable ".\\sharedV.lvlib\\Encoder_Swing"() -> (w349:dbl)  [unwired: 1 in, 1 out]
    n142 = shared-variable ".\\sharedV.lvlib\\Encoder_Boom"() -> (w348:dbl)  [unwired: 1 in, 1 out]
    n143 = shared-variable ".\\sharedV.lvlib\\Encoder_Stick"() -> (w347:dbl)  [unwired: 1 in, 1 out]
    n144 = shared-variable ".\\sharedV.lvlib\\Referenc_Pressure"() -> (w353:dbl)  [unwired: 1 in, 1 out]
    n145 = shared-variable ".\\sharedV.lvlib\\Swing_Joint_Pi"() -> (w365:dbl)  [unwired: 1 in, 1 out]
    n146 = shared-variable ".\\sharedV.lvlib\\Boom_Joint_Pi"() -> (w363:dbl)  [unwired: 1 in, 1 out]
    n147 = shared-variable ".\\sharedV.lvlib\\Stick_Joint_Pi"() -> (w362:dbl)  [unwired: 1 in, 1 out]
    n148 = shared-variable ".\\sharedV.lvlib\\Swing_Joint_Po"() -> (w361:dbl)  [unwired: 1 in, 1 out]
    n149 = shared-variable ".\\sharedV.lvlib\\Boom_Joint_Po"() -> (w360:dbl)  [unwired: 1 in, 1 out]
    n150 = shared-variable ".\\sharedV.lvlib\\Stick_Joint_Po"() -> (w345:dbl)  [unwired: 1 in, 1 out]
    n151 = shared-variable ".\\sharedV.lvlib\\Sample_Time"() -> (w346:dbl)  [unwired: 1 in, 1 out]
    n152 = shared-variable ".\\sharedV.lvlib\\Desired_Tol_Swing"() -> (w337:dbl[])  [unwired: 1 in, 1 out]
    n153 = shared-variable ".\\sharedV.lvlib\\Desired_Tol_Boom"() -> (w336:dbl[])  [unwired: 1 in, 1 out]
    n154 = shared-variable ".\\sharedV.lvlib\\Desired_Tol_Stick"() -> (w335:dbl[])  [unwired: 1 in, 1 out]
    n155 = shared-variable ".\\sharedV.lvlib\\Desired_q_Boom"() -> (w331:dbl)  [unwired: 1 in, 1 out]
    n156 = shared-variable ".\\sharedV.lvlib\\Desired_q_Swing"() -> (w330:dbl)  [unwired: 1 in, 1 out]
    n157 = shared-variable ".\\sharedV.lvlib\\Desired_q_Stick"() -> (w332:dbl)  [unwired: 1 in, 1 out]
    n158 = shared-variable ".\\sharedV.lvlib\\Sample_Time"() -> (w243:dbl)  [unwired: 1 in, 1 out]
    n159 = Tick Count (ms) ("时间计数器")() -> (millisecond timer value=w232:u32)
    n160 = Multiply ("乘")(x=1e-08, y="gamma_d2(E-8)") -> (x*y=w325:dbl[])
    n161 = Divide ("除")(x=w232, y=u32 1000) -> (x/y=w240:dbl)
    n162 = expression code="(x/180.0)*pi"(w349) -> (w372:dbl)
    n163 = expression code="(x/180.0)*pi"(w348) -> (w334:dbl)
    n164 = expression code="(x/180.0)*pi"(w347) -> (w333:dbl)
    n165 = Multiply ("乘")(x=w243, y=w233) -> (x*y=w242:dbl)
    n166 = expression code="(x/180.0)*pi"(w371) -> (w370:dbl)
    n167 = expression code="(x/180.0)*pi"(w368) -> (w369:dbl)
    n168 = expression code="(x/180.0)*pi"(w367) -> (w366:dbl)
    n169 = Multiply ("乘")(x=w350, y=w365) -> (x*y=w364:dbl)
    n170 = Multiply ("乘")(x=w350, y=w363) -> (x*y=w355:dbl)
    n171 = Multiply ("乘")(x=w350, y=w362) -> (x*y=w356:dbl)
    n172 = Multiply ("乘")(x=w350, y=w361) -> (x*y=w357:dbl)
    n173 = Multiply ("乘")(x=w350, y=w360) -> (x*y=w358:dbl)
    n174 = Multiply ("乘")(x=w350, y=w345) -> (x*y=w359:dbl)
    n175 = Multiply ("乘")(x=w350, y=w353) -> (x*y=w354:dbl)
    n176 = Subtract ("减")(x=w240, y=w242) -> (x-y=w236:dbl)
    n177 = feedback #3 ("反馈节点")(0.0) -> (w235:dbl)
    n178 = feedback-in #3(w236) -> ()
    n179 = Subtract ("减")(x=w236, y=w235) -> (x-y=w239:dbl)
    n180 = Less? ("小于？")(x=w239, y=1e-05) -> (x < y?=→"No error 3":bool)
    n181 = Multiply ("乘")(x=1e-08, y="K3(E-8)") -> (x*y=w322:dbl[])
    n182 = feedback #4 "q_f"(w275) -> (w277:dbl[])
    n183 = feedback #5 "q_dot_f"(w275) -> (w276:dbl[])
    n184 = feedback #6 "Theta_F_Boom"(w275) -> (w300:dbl[])
    n185 = feedback #7 "Theta_Q_Boom"(w275) -> (w299:dbl[])
    n186 = feedback #8 "Theta_Q_Swing"(w275) -> (w302:dbl[])
    n187 = feedback #9 "Theta_Q_Stick"(w305) -> (w306:dbl[])
    n188 = feedback #10 "Gamma_1_Swing"(w259) -> (w272:dbl)
    n189 = feedback #11 "Gamma_2_Swing"(w260) -> (w270:dbl)
    n190 = feedback #12 "Gamma_1_Boom"(w259) -> (w268:dbl)
    n191 = feedback #13 "Gamma_2_Boom"(w260) -> (w266:dbl)
    n192 = feedback #14 "Gamma_1"(w259) -> (w264:dbl)
    n193 = feedback #15 "Gamma_2"(w260) -> (w262:dbl)
    n194 = feedback #16 "Theta_F_Swing"(w275) -> (w304:dbl[])
    n195 = feedback #17 "Theta_F_Stick"(w307) -> (w308:dbl[])
    n196 = Multiply ("乘")(x=1e-08, y="Theta_s2_init(E-8)") -> (x*y=w315:dbl[])
    n197 = feedback #18 "d1_hat"(w275) -> (w321:dbl[])
    n198 = feedback #19 "d2_hat"(w275) -> (w319:dbl[])
    n199 = feedback #20 "X1_f"(w310) -> (w314:dbl[])
    n200 = feedback #21 "X2_f"(w309) -> (w313:dbl[])
    n201 = mathscript code="%%Author : Manzhi Qi\nq = [q1, q2, q3]';\n% 期望轨迹数据重组  rad\n% qd           =  [Desired_Swing(1), Desired_Boom(1), Desired_Stick(1)]';\nqd           =  [Desired_q_Swing, Desired_q_Boom, Desired_q_Stick]' * pi / 180;\nqd_dot     =  [Desired_Swing(2), Desired_Boom(2), Desired_Stick(2)]';\nqd_ddot   =  [Desired_Swing(3), Desired_Boom(3), Desired_Stick(3)]';\nqd_dddot =  [Desired_Swing(4), Desired_Boom(4), Desired_Stick(4)]';\n% 控制三角形夹角 rad\nalpha = [alpha1, alpha2, alpha3]'; \n\n% 液压缸压力 Pa\nPi = [pi1, pi2, pi3]';\nPo = [po1, po2, po3]';\n\n%% ----------------------硬件参数----------------------\ndeg2rad = 2*pi/360;                             % 角度制转弧度制\nmm2m = 1e-3;                                    % 毫米制转米制\ng = 9.8;                                        % 重力加速度\nAB = [230, 261, 245]' .* mm2m;             % R3*1：控制三角形邻边A\nBC = [46,   60,  50]' .* mm2m;             % R3*1：控制三角形邻边B\nx0Total = [190, 207, 202]' .* mm2m;        % 液压缸的初始长度（x=0）\n%D1 = [32, 50, 40]' .* mm2m;                 % 液压缸直径\n%D2 = [16, 25, 16]' .* mm2m;                 % 液压缸伸出杆直径\nD1 = [50, 50, 50]' .* mm2m;                 % 液压缸直径\nD2 = [25, 25, 25]' .* mm2m;                 % 液压缸伸出杆直径\nxmax = [80, 104, 82]' .* 1e-3;              % 液压缸总行程长度\nlength1_pipeline = [500, 500+300, 500+300+100]' .* mm2m;   % 无杆腔油管长度\nlength2_pipeline = [600, 600+200, 600+200+400]' .* mm2m;   % 有杆腔油管长度\nD_pipeline = 1/6 * 0.0254;                      % 油管直径\nL = [101.1, 605, 284.4]' .* mm2m;            % 臂长\nm = [6, 5.5, 3.3]'  + [1, 2, 0]';                      % 连杆质量+液压缸质量\nr = L/2;                                                                    % 质心位置\nIx = [13826,  14322,  19924]' .* mm2m .* mm2m;                        \nIy = [30072, 614730, 138744]' .* mm2m .* mm2m;                       \nIz = [21003, 609974, 144768]' .* mm2m .* mm2m;                       \n% q = [0,10/57,60/57,40/57];                                                \n% qd = [0,0,0.1,1];                                                      \nIx1 = Ix(1); Ix2 = Ix(2); Ix3 = Ix(3);\nIy1 = Iy(1); Iy2 = Iy(2); Iy3 = Iy(3);\nIz1 = Iz(1); Iz2 = Iz(2); Iz3 = Iz(3);\nm1 = m(1); m2 = m(2); m3 = m(3); \nr1 = r(1); r2 = r(2); r3 = r(3); \nL1 = L(1); L2 = L(2); L3 = L(3); \n\nfor ii = 1:3\n  xNowTotal(ii) = sqrt(AB(ii)^2 + BC(ii)^2 - 2*AB(ii)*BC(ii)*cos(alpha(ii)));           \t%控制三角形中关节角对应边长\nend\nxNowTotal = xNowTotal(:);\nJ_h = diag((AB .* BC .* sin(alpha)) ./ xNowTotal);\ninv_J_h = diag(xNowTotal./ (AB .* BC .* sin(alpha)));\n% 液压相关\nA_pipeline = 0.25*pi*D_pipeline^2;        \t        % 油管面积\nAi = 0.25*pi*D1.^2;                                 % 无杆腔面积\nAo = Ai - 0.25*pi*D2.^2;                      \t    % 有杆腔面积\nVh1 = A_pipeline .* length1_pipeline;               % 无杆腔油管油液体积\nVh2 = A_pipeline.*length2_pipeline + xmax.*Ao;      % 有杆腔油管油液体积\nxL = xNowTotal - x0Total;                           % 液压缸位移\nVi = Vh1 + Ai.*xL;                                  % 无杆腔油液总体积\nVo = Vh2 - Ao.*xL;                                  % 有杆腔油液总体积\nA_Q = Ai.^2./Vi + Ao.^2./Vo;\nB_Q = Ai ./ Vi;\nC_Q = Ao ./ Vo;\n\n% 二阶微分滤波求q_dot q_ddot.................\nq_dot_f = q_dot_f(:);\nq_f = q_f(:);\nq_dot = q_dot_f;\nwn = 100; % 原先是100，为了减少相位滞后，应当尽可能大\nepsilon = 0.707;\nq_ddot_f = wn^2*q - 2*epsilon*wn*q_dot_f - wn^2*q_f;\nq_dot_f_next = q_dot_f + q_ddot_f*ts;\nq_f_next = q_f + q_dot_f.*ts;\n\n%%\nq1d = q_dot(1);  q2d = q_dot(2);  q3d = q_dot(3); \nM =...\n[Ix2/2 + Ix3/2 + Iy2/2 + Iy3/2 + Iz1 - (Ix3*cos(2*q2 + 2*q3))/2 + (Iy3*cos(2*q2 + 2*q3))/2 + L1^2*m2 + L1^2*m3 + (L2^2*m3)/2 + (L3^2*m3)/2 + m1*r1^2 + (m2*r2^2)/2 - (Ix2*cos(2*q2))/2 + (Iy2*cos(2*q2))/2 + (L2^2*m3*cos(2*q2))/2 + (m2*r2^2*cos(2*q2))/2 + (L3^2*m3*cos(2*q2 + 2*q3))/2 + 2*L1*L3*m3*cos(q2 + q3) + 2*L1*L2*m3*cos(q2) + L2*L3*m3*cos(q3) + 2*L1*m2*r2*cos(q2) + L2*L3*m3*cos(2*q2 + q3),                                                            0,                                0;\n                                                                                                                                                                                                                                                                                                                                                                                                        0, m3*L2^2 + 2*m3*cos(q3)*L2*r3 + m2*r2^2 + m3*r3^2 + Iz2 + Iz3, m3*r3^2 + L2*m3*cos(q3)*r3 + Iz3;\n                                                                                                                                                                                                                                                                                                                                                                                                        0,                             m3*r3^2 + L2*m3*cos(q3)*r3 + Iz3,                    m3*r3^2 + Iz3];\n\nC =...\n[- q2d*((m3*sin(2*q2)*L2^2)/2 + m3*sin(2*q2 + q3)*L2*L3 + L1*m3*sin(q2)*L2 + (m3*sin(2*q2 + 2*q3)*L3^2)/2 + L1*m3*sin(q2 + q3)*L3 + (m2*sin(2*q2)*r2^2)/2 + L1*m2*sin(q2)*r2 - (Ix3*sin(2*q2 + 2*q3))/2 + (Iy3*sin(2*q2 + 2*q3))/2 - (Ix2*sin(2*q2))/2 + (Iy2*sin(2*q2))/2) - q3d*((Iy3*sin(2*q2 + 2*q3))/2 - (Ix3*sin(2*q2 + 2*q3))/2 + (L3^2*m3*sin(2*q2 + 2*q3))/2 + L1*L3*m3*sin(q2 + q3) + (L2*L3*m3*sin(q3))/2 + (L2*L3*m3*sin(2*q2 + q3))/2),  -q1d*((m3*sin(2*q2)*L2^2)/2 + m3*sin(2*q2 + q3)*L2*L3 + L1*m3*sin(q2)*L2 + (m3*sin(2*q2 + 2*q3)*L3^2)/2 + L1*m3*sin(q2 + q3)*L3 + (m2*sin(2*q2)*r2^2)/2 + L1*m2*sin(q2)*r2 - (Ix3*sin(2*q2 + 2*q3))/2 + (Iy3*sin(2*q2 + 2*q3))/2 - (Ix2*sin(2*q2))/2 + (Iy2*sin(2*q2))/2),  -q1d*((Iy3*sin(2*q2 + 2*q3))/2 - (Ix3*sin(2*q2 + 2*q3))/2 + (L3^2*m3*sin(2*q2 + 2*q3))/2 + L1*L3*m3*sin(q2 + q3) + (L2*L3*m3*sin(q3))/2 + (L2*L3*m3*sin(2*q2 + q3))/2);\n                                                                                                                                                                           q1d*((m3*sin(2*q2)*L2^2)/2 + m3*sin(2*q2 + q3)*L2*L3 + L1*m3*sin(q2)*L2 + (m3*sin(2*q2 + 2*q3)*L3^2)/2 + L1*m3*sin(q2 + q3)*L3 + (m2*sin(2*q2)*r2^2)/2 + L1*m2*sin(q2)*r2 - (Ix3*sin(2*q2 + 2*q3))/2 + (Iy3*sin(2*q2 + 2*q3))/2 - (Ix2*sin(2*q2))/2 + (Iy2*sin(2*q2))/2),                                                                                                                                                                                                                                                      -L2*m3*q3d*r3*sin(q3),                                                                                                                                           -L2*m3*r3*sin(q3)*(q2d + q3d);\n                                                                                                                                                                                                                                                                              q1d*((Iy3*sin(2*q2 + 2*q3))/2 - (Ix3*sin(2*q2 + 2*q3))/2 + (L3^2*m3*sin(2*q2 + 2*q3))/2 + L1*L3*m3*sin(q2 + q3) + (L2*L3*m3*sin(q3))/2 + (L2*L3*m3*sin(2*q2 + q3))/2),                                                                                                                                                                                                                                                       L2*m3*q2d*r3*sin(q3),                                                                                                                                                                       0;];\n\nG = [                                                    0;\n    g*(m2*r2*cos(q2) + m3*r3*cos(q2 + q3) + L2*m3*cos(q2));\n                                      g*m3*r3*cos(q2 + q3);] ;\n\n\nq1d_d = qd_dot(1);  q2d_d = qd_dot(2);  q3d_d = qd_dot(3); \nq1_d = qd(1);  q2_d = qd(2);  q3_d = qd(3); \nM_d =...\n[Ix2/2 + Ix3/2 + Iy2/2 + Iy3/2 + Iz1 - (Ix3*cos(2*q2_d + 2*q3_d))/2 + (Iy3*cos(2*q2_d + 2*q3_d))/2 + L1^2*m2 + L1^2*m3 + (L2^2*m3)/2 + (L3^2*m3)/2 + m1*r1^2 + (m2*r2^2)/2 - (Ix2*cos(2*q2_d))/2 + (Iy2*cos(2*q2_d))/2 + (L2^2*m3*cos(2*q2_d))/2 + (m2*r2^2*cos(2*q2_d))/2 + (L3^2*m3*cos(2*q2_d + 2*q3_d))/2 + 2*L1*L3*m3*cos(q2_d + q3_d) + 2*L1*L2*m3*cos(q2_d) + L2*L3*m3*cos(q3_d) + 2*L1*m2*r2*cos(q2_d) + L2*L3*m3*cos(2*q2_d + q3_d),                                                            0,                                0;\n                                                                                                                                                                                                                                                                                                                                                                                                        0, m3*L2^2 + 2*m3*cos(q3_d)*L2*r3 + m2*r2^2 + m3*r3^2 + Iz2 + Iz3, m3*r3^2 + L2*m3*cos(q3_d)*r3 + Iz3;\n                                                                                                                                                                                                                                                                                                                                                                                                        0,                             m3*r3^2 + L2*m3*cos(q3_d)*r3 + Iz3,                    m3*r3^2 + Iz3];\n\nC_d =...\n[- q2d_d*((m3*sin(2*q2_d)*L2^2)/2 + m3*sin(2*q2_d + q3_d)*L2*L3 + L1*m3*sin(q2_d)*L2 + (m3*sin(2*q2_d + 2*q3_d)*L3^2)/2 + L1*m3*sin(q2_d + q3_d)*L3 + (m2*sin(2*q2_d)*r2^2)/2 + L1*m2*sin(q2_d)*r2 - (Ix3*sin(2*q2_d + 2*q3_d))/2 + (Iy3*sin(2*q2_d + 2*q3_d))/2 - (Ix2*sin(2*q2_d))/2 + (Iy2*sin(2*q2_d))/2) - q3d_d*((Iy3*sin(2*q2_d + 2*q3_d))/2 - (Ix3*sin(2*q2_d + 2*q3_d))/2 + (L3^2*m3*sin(2*q2_d + 2*q3_d))/2 + L1*L3*m3*sin(q2_d + q3_d) + (L2*L3*m3*sin(q3_d))/2 + (L2*L3*m3*sin(2*q2_d + q3_d))/2),  -q1d_d*((m3*sin(2*q2_d)*L2^2)/2 + m3*sin(2*q2_d + q3_d)*L2*L3 + L1*m3*sin(q2_d)*L2 + (m3*sin(2*q2_d + 2*q3_d)*L3^2)/2 + L1*m3*sin(q2_d + q3_d)*L3 + (m2*sin(2*q2_d)*r2^2)/2 + L1*m2*sin(q2_d)*r2 - (Ix3*sin(2*q2_d + 2*q3_d))/2 + (Iy3*sin(2*q2_d + 2*q3_d))/2 - (Ix2*sin(2*q2_d))/2 + (Iy2*sin(2*q2_d))/2),  -q1d_d*((Iy3*sin(2*q2_d + 2*q3_d))/2 - (Ix3*sin(2*q2_d + 2*q3_d))/2 + (L3^2*m3*sin(2*q2_d + 2*q3_d))/2 + L1*L3*m3*sin(q2_d + q3_d) + (L2*L3*m3*sin(q3_d))/2 + (L2*L3*m3*sin(2*q2_d + q3_d))/2);\n                                                                                                                                                                           q1d_d*((m3*sin(2*q2_d)*L2^2)/2 + m3*sin(2*q2_d + q3_d)*L2*L3 + L1*m3*sin(q2_d)*L2 + (m3*sin(2*q2_d + 2*q3_d)*L3^2)/2 + L1*m3*sin(q2_d + q3_d)*L3 + (m2*sin(2*q2_d)*r2^2)/2 + L1*m2*sin(q2_d)*r2 - (Ix3*sin(2*q2_d + 2*q3_d))/2 + (Iy3*sin(2*q2_d + 2*q3_d))/2 - (Ix2*sin(2*q2_d))/2 + (Iy2*sin(2*q2_d))/2),                                                                                                                                                                                                                                                      -L2*m3*q3d_d*r3*sin(q3_d),                                                                                                                                           -L2*m3*r3*sin(q3_d)*(q2d_d + q3d_d);\n                                                                                                                                                                                                                                                                              q1d_d*((Iy3*sin(2*q2_d + 2*q3_d))/2 - (Ix3*sin(2*q2_d + 2*q3_d))/2 + (L3^2*m3*sin(2*q2_d + 2*q3_d))/2 + L1*L3*m3*sin(q2_d + q3_d) + (L2*L3*m3*sin(q3_d))/2 + (L2*L3*m3*sin(2*q2_d + q3_d))/2),                                                                                                                                                                                                                                                       L2*m3*q2d_d*r3*sin(q3_d),                                                                                                                                                                       0;];\n\nG_d = [                                                    0;\n    g*(m2*r2*cos(q2_d) + m3*r3*cos(q2_d + q3_d) + L2*m3*cos(q2_d));\n                                      g*m3*r3*cos(q2_d + q3_d);] ;\n\n\n\n\n%% Update\nTheta_s1_init = Theta_s1_init(:);\nTheta_s2_init = Theta_s2_init(:);\n%% 预处理\ntheta_hat1 = zeros(3,1);\ntheta_hat2 = zeros(3,1);\ntheta_hat3 = zeros(3,1);\ntheta_hat4 = zeros(3,1);\ntheta_hat5 = zeros(3,1);\ntheta_hat6 = zeros(3,1);\n\ntheta_hat1 (1) = Theta_Swing_F_hat (1); % fv\ntheta_hat2 (1) = Theta_Swing_F_hat (2); % fc\ntheta_hat3 (1) = Theta_Swing_F_hat (3); % D_Fn\ntheta_hat4 (1) = Theta_Swing_Q_hat (1); % 1/beta_e\ntheta_hat5 (1) = Theta_Swing_Q_hat (2); % D_Qin\ntheta_hat6 (1) = Theta_Swing_Q_hat (3); % D_Qon\n\ntheta_hat1 (2) = Theta_Boom_F_hat (1);\ntheta_hat2 (2) = Theta_Boom_F_hat (2);\ntheta_hat3 (2) = Theta_Boom_F_hat (3);\ntheta_hat4 (2) = Theta_Boom_Q_hat (1);\ntheta_hat5 (2) = Theta_Boom_Q_hat (2);\ntheta_hat6 (2) = Theta_Boom_Q_hat (3);\n\ntheta_hat1 (3) = Theta_Stick_F_hat (1);\ntheta_hat2 (3) = Theta_Stick_F_hat (2);\ntheta_hat3 (3) = Theta_Stick_F_hat (3);\ntheta_hat4 (3) = Theta_Stick_Q_hat (1);\ntheta_hat5 (3) = Theta_Stick_Q_hat (2);\ntheta_hat6 (3) = Theta_Stick_Q_hat (3);\n\n\n%% step1\nK1 = K1(:);\nK2 = K2(:);\nK3 = K3(:);\ne1 = q - qd;\ne1_dot = q_dot - qd_dot;\nqeq_dot = qd_dot - K1.*e1;\nqeq_ddot = qd_ddot - K1.*e1_dot;\ne2 = q_dot - qeq_dot;\nS_qdot = 2/pi*atan(900*q_dot);   \nSd_qdot = 2/pi*atan(900*qd_dot);   \n\nFLda1 = inv_J_h * (M_d * qeq_dot + C_d * qd_dot + G_d + theta_hat1 .* qd_dot + theta_hat2 .* Sd_qdot - theta_hat3);\nFLds1 = - inv_J_h * K2 .* e2;\nFLda2 = - inv_J_h * d1hat(:);\nFLds2 = 0;\n\nFLd = FLda1* sw_FLda1 + FLda2  + FLds1 + FLds2;\nFL = Pi.*Ai - Po.*Ao; \ne3 = FL - FLd;\n%% step2\nFLdc_dot = zeros(3,1);\n\n% QLda1 = J_h*A_Q*q_dot - B_Q*theta_hat4 - C_Q*theta_hat5 + FLdc_dot*theta_hat6 + Upsilon_Q;\nw1 = w1( : ) ;\nw2 = w2 ( : ); \nomega = w1 ./ w2 ;\n\nQLda1 = J_h*diag(A_Q) * qd_dot + diag(FLdc_dot) * theta_hat4 - diag(B_Q) * theta_hat5 - diag(C_Q) * theta_hat6 ;\nQLda2 = -d2hat( : );\nQLds1 = -K3 .* e3;     \nY_Q = -J_h * omega .* e2 * sw_Y_Q;                                    \nQLd = QLda1 * sw_QLda1 + QLda2  +  QLds1  + Y_Q; \ne2_e3 = e2./e3;\n\n\n%% ----------------------Filtering----------------------\ntau_f = 0.006 ;\ntemp_A  = [q_dot ; S_qdot ; - ones(3,1) ; B_Q ;  C_Q ; (J_h * FL + C' * q_dot - G) ] ;  % Normal Filiter var R 18*1\ntemp_B = [FL ; M * q_dot ];  % first-order Filiter var  R 6*1\n% Normal Filiter\nX1_f_next = (temp_A - X1_f( : )) / tau_f * ts + X1_f( : );\n% first-order Filiter\nX2_f_next = (temp_B - X2_f( : )) / tau_f * ts + X2_f( : ) ;\ntemp_B_dot  = (temp_B - X2_f( : )) / tau_f ;\n\nfilter_FL_dot = temp_B_dot(1 : 3);\nfilter_P_dot = temp_B_dot(4 : 6);\n\nA_f = X1_f_next(16 : 18);\nB_Q_f = X1_f_next ( 10 : 12 ) ;\nC_Q_f = X1_f_next ( 13 : 15 ) ;\nu1f_phi = filter_P_dot - A_f;\nu2f_phi = QLd - J_h * diag(A_Q) * q_dot; \n\nphi1f = reshape( X1_f_next ( 1 : 9 ) , 3 , 3 ) ;   % Arrange by column q_dot / S_qdot / - ones(3,1)\ntemp =  [ -filter_FL_dot ; B_Q_f ; C_Q_f ];\nphi2f = reshape( temp  , 3 , 3 ) ; % Arrange by column -FL_dot / B_Q / C_Q\n\n\n%%  ----------------------Theta_Updata----------------------\nF_Phi_Swing = phi1f ( 1 , : )';\nQ_Phi_Swing = phi2f ( 1 , : )';\nF_Phi_Boom= phi1f ( 2 , : )';\nQ_Phi_Boom = phi2f ( 2 , : )';\nF_Phi_Stick = phi1f ( 3 , : )';\nQ_Phi_Stick = phi2f ( 3 , : )';\n%Theta_Stick_hat = zeros(3,1);\nTheta_Swing_F_hat = Theta_Swing_F_hat( : );\nTheta_Swing_Q_hat = Theta_Swing_Q_hat( : );\nTheta_Boom_F_hat = Theta_Boom_F_hat( : );\nTheta_Boom_Q_hat = Theta_Boom_Q_hat( : );\nTheta_Stick_F_hat = Theta_Stick_F_hat( : );\nTheta_Stick_Q_hat = Theta_Stick_Q_hat( : );\nv1 = 0.1;\nv2 = 0.1;\n\n% Calculate estimation errors Epsilon\nEpsilon_1 = zeros(3, 1);\nEpsilon_2 = zeros(3, 1);\nEpsilon_1(1) = -F_Phi_Swing' * Theta_Swing_F_hat - u1f_phi(1);   % Swing\nEpsilon_1(2) = -F_Phi_Boom' * Theta_Boom_F_hat - u1f_phi(2);     % Boom\nEpsilon_1(3) = -F_Phi_Stick' * Theta_Stick_F_hat - u1f_phi(3);   % Stick\n\nEpsilon_2(1) = -Q_Phi_Swing' * Theta_Swing_Q_hat - u2f_phi(1);   % Swing\nEpsilon_2(2) = -Q_Phi_Boom' * Theta_Boom_Q_hat - u2f_phi(2);     % Boom\nEpsilon_2(3) = -Q_Phi_Stick' * Theta_Stick_Q_hat - u2f_phi(3);   % Stick\n\n% Calculate xi\nxi_1 = zeros(3, 1);\nxi_2 = zeros(3, 1);\nxi_1(1) = 1 / (1 + v1 * F_Phi_Swing' * Gamma_1_Swing * F_Phi_Swing);  % Swing\nxi_1(2) = 1 / (1 + v1 * F_Phi_Boom' * Gamma_1_Boom * F_Phi_Boom);     % Boom\nxi_1(3) = 1 / (1 + v1 * F_Phi_Stick' * Gamma_1 * F_Phi_Stick);        % Stick\n\nxi_2(1) = 1 / (1 + v2 * Q_Phi_Swing' * Gamma_2_Swing * Q_Phi_Swing);  % Swing\nxi_2(2) = 1 / (1 + v2 * Q_Phi_Boom' * Gamma_2_Boom * Q_Phi_Boom);     % Boom\nxi_2(3) = 1 / (1 + v2 * Q_Phi_Stick' * Gamma_2 * Q_Phi_Stick);        % Stick\n\n% Since tau vectors might have different dimensions, store them separately\ntau_1_Swing = xi_1(1) * F_Phi_Swing * Epsilon_1(1);  % Swing\ntau_1_Boom = xi_1(2) * F_Phi_Boom * Epsilon_1(2);    % Boom\ntau_1_Stick = xi_1(3) * F_Phi_Stick * Epsilon_1(3);  % Stick\n\ntau_2_Swing = xi_2(1) * Q_Phi_Swing * Epsilon_2(1);  % Swing\ntau_2_Boom = xi_2(2) * Q_Phi_Boom * Epsilon_2(2);    % Boom\ntau_2_Stick = xi_2(3) * Q_Phi_Stick * Epsilon_2(3);  % Stick\n\n% Calculate derivatives of Theta_hat\nTheta_Swing_F_hat_dot = Gamma_1_Swing * tau_1_Swing;  % Swing\nTheta_Boom_F_hat_dot = Gamma_1_Boom * tau_1_Boom;     % Boom\nTheta_Stick_F_hat_dot = Gamma_1 * tau_1_Stick;        % Stick\n\nTheta_Swing_Q_hat_dot = Gamma_2_Swing * tau_2_Swing;  % Swing\nTheta_Boom_Q_hat_dot = Gamma_2_Boom * tau_2_Boom;     % Boom\nTheta_Stick_Q_hat_dot = Gamma_2 * tau_2_Stick;        % Stick\n\n% Calculate Theta_hat for next time step\nTheta_Swing_F_hat_next = Theta_Swing_F_hat_dot * ts + Theta_Swing_F_hat;  % Swing\nTheta_Boom_F_hat_next = Theta_Boom_F_hat_dot * ts + Theta_Boom_F_hat;     % Boom\nTheta_Stick_F_hat_next = Theta_Stick_F_hat_dot * ts + Theta_Stick_F_hat;  % Stick\n\nTheta_Swing_Q_hat_next = Theta_Swing_Q_hat_dot * ts + Theta_Swing_Q_hat;  % Swing\nTheta_Boom_Q_hat_next = Theta_Boom_Q_hat_dot * ts + Theta_Boom_Q_hat;     % Boom\nTheta_Stick_Q_hat_next = Theta_Stick_Q_hat_dot * ts + Theta_Stick_Q_hat;  % Stick\n\n% Parameter limits\nTheta_Swing_Max = [2000, 20000, 200, 1/(2e8), 1e-5, 1e-5];  % fv fc D_Fn D_Qin D_Qon 1/beta\nTheta_Swing_Min = [10,      10,     -200, 1/(1.25e9), -1e-5, -1e-5];\nTheta_Boom_Max = [2000, 20000, 200, 1/(2e8), 1e-5, 1e-5];  % fv fc D_Fn D_Qin D_Qon 1/beta\nTheta_Boom_Min = [10,      10,     -200, 1/(1.25e9), -1e-5, -1e-5];\nTheta_Stick_Max = [2000, 20000, 200, 1/(2e8), 1e-5, 1e-5];  % fv fc D_Fn D_Qin D_Qon 1/beta\nTheta_Stick_Min = [10,      10,     -200, 1/(1.25e9), -1e-5, -1e-5];\n\nTheta_Swing_Max = [2000, 20000, 200, 1/(2e8), 1e-1, 1e-1];  % fv fc D_Fn D_Qin D_Qon 1/beta\nTheta_Swing_Min = [10,      10,     -200, 1/(1.25e9), -1e-1, -1e-1];\n\nTheta_Boom_Max = [2000, 20000, 200, 1/(2e8), 1e-1, 1e-1];  % fv fc D_Fn D_Qin D_Qon 1/beta\nTheta_Boom_Min = [10,      10,     -200, 1/(1.25e9), -1e-1, -1e-1];\n\nTheta_Stick_Max = [2000, 20000, 200, 1/(2e8), 1e-1, 1e-1];  % fv fc D_Fn D_Qin D_Qon 1/beta\nTheta_Stick_Min = [10,      10,     -200, 1/(1.25e9), -1e-1, -1e-1];\n\n% Apply parameter limits\nfor idx = 1:3\n    %Swing\n    Theta_Swing_F_hat_next(idx) = min(max(Theta_Swing_F_hat_next(idx), Theta_Swing_Min(idx)), Theta_Swing_Max(idx));\n    Theta_Swing_Q_hat_next(idx) = min(max(Theta_Swing_Q_hat_next(idx), Theta_Swing_Min(idx + 3)), Theta_Swing_Max(idx + 3));\n    \n    %Boom\n    Theta_Boom_F_hat_next(idx) = min(max(Theta_Boom_F_hat_next(idx), Theta_Boom_Min(idx)), Theta_Boom_Max(idx));\n    Theta_Boom_Q_hat_next(idx) = min(max(Theta_Boom_Q_hat_next(idx), Theta_Boom_Min(idx + 3)), Theta_Boom_Max(idx + 3));\n    \n    %Stick\n    Theta_Stick_F_hat_next(idx) = min(max(Theta_Stick_F_hat_next(idx), Theta_Stick_Min(idx)), Theta_Stick_Max(idx));\n    Theta_Stick_Q_hat_next(idx) = min(max(Theta_Stick_Q_hat_next(idx), Theta_Stick_Min(idx + 3)), Theta_Stick_Max(idx + 3));\nend\n\n\nif  Use_Preset_Theta == 1\n    Theta_Swing_F_hat_next = [Theta_s1_init(1);Theta_s1_init(4);Theta_s1_init(7)];\n    Theta_Boom_F_hat_next = [Theta_s1_init(2);Theta_s1_init(5);Theta_s1_init(8)];\n    Theta_Stick_F_hat_next = [Theta_s1_init(3);Theta_s1_init(6);Theta_s1_init(9)];\n    Theta_Swing_Q_hat_next = [Theta_s2_init(1);Theta_s2_init(4);Theta_s2_init(7)];\n    Theta_Boom_Q_hat_next = [Theta_s2_init(2);Theta_s2_init(5);Theta_s2_init(8)];\n    Theta_Stick_Q_hat_next = [Theta_s2_init(3);Theta_s2_init(6);Theta_s2_init(9)];\nend\n\n\nif  Stop_Theta_Update == 1\n    Theta_Swing_F_hat_next = Theta_Swing_F_hat;\n    Theta_Boom_F_hat_next = Theta_Boom_F_hat;\n    Theta_Stick_F_hat_next = Theta_Stick_F_hat;\n    Theta_Swing_Q_hat_next = Theta_Swing_Q_hat;\n    Theta_Boom_Q_hat_next = Theta_Boom_Q_hat;\n    Theta_Stick_Q_hat_next = Theta_Stick_Q_hat;\nend\n%% ----------------------Gamma_Update----------------------\n% Update rates\nalpha_1 = 0.2;\nalpha_2 = 0.2;\n\n% Calculate Gamma derivatives\nGamma_1_Swing_dot = alpha_1 * Gamma_1_Swing - xi_1(1) * Gamma_1_Swing * F_Phi_Swing' * F_Phi_Swing * Gamma_1_Swing;\nGamma_1_Boom_dot = alpha_1 * Gamma_1_Boom - xi_1(2) * Gamma_1_Boom * F_Phi_Boom' * F_Phi_Boom * Gamma_1_Boom;\nGamma_1_dot = alpha_1 * Gamma_1 - xi_1(3) * Gamma_1 * F_Phi_Stick' * F_Phi_Stick * Gamma_1;\n\nGamma_2_Swing_dot = alpha_2 * Gamma_2_Swing - xi_2(1) * Gamma_2_Swing * Q_Phi_Swing' * Q_Phi_Swing * Gamma_2_Swing;\nGamma_2_Boom_dot = alpha_2 * Gamma_2_Boom - xi_2(2) * Gamma_2_Boom * Q_Phi_Boom' * Q_Phi_Boom * Gamma_2_Boom;\nGamma_2_dot = alpha_2 * Gamma_2 - xi_2(3) * Gamma_2 * Q_Phi_Stick' * Q_Phi_Stick * Gamma_2;\n\n% Update Gamma matrices\nGamma_1_Swing_next = Gamma_1_Swing_dot * ts + Gamma_1_Swing;\nGamma_1_Boom_next = Gamma_1_Boom_dot * ts + Gamma_1_Boom;\nGamma_1_next = Gamma_1_dot * ts + Gamma_1;\n\nGamma_2_Swing_next = Gamma_2_Swing_dot * ts + Gamma_2_Swing;\nGamma_2_Boom_next = Gamma_2_Boom_dot * ts + Gamma_2_Boom;\nGamma_2_next = Gamma_2_dot * ts + Gamma_2;\n\n% Gamma limits\nGamma_1_Max = [1000, 1000, 1000];\nGamma_1_Min = -Gamma_1_Max;\nGamma_2_Max = [1e-1, 1e-3, 1e-3];\nGamma_2_Min = -Gamma_2_Max;\n\n% Apply Gamma limits\nfor idx = 1:3\n    % Swing\n    Gamma_1_Swing_next  = min(max(Gamma_1_Swing_next , Gamma_1_Min(idx)), Gamma_1_Max(idx));\n    Gamma_2_Swing_next  = min(max(Gamma_2_Swing_next , Gamma_2_Min(idx)), Gamma_2_Max(idx));\n    \n    % Boom\n    Gamma_1_Boom_next  = min(max(Gamma_1_Boom_next , Gamma_1_Min(idx)), Gamma_1_Max(idx));\n    Gamma_2_Boom_next  = min(max(Gamma_2_Boom_next , Gamma_2_Min(idx)), Gamma_2_Max(idx));\n    \n    % Stick\n    Gamma_1_next = min(max(Gamma_1_next , Gamma_1_Min(idx)), Gamma_1_Max(idx));\n    Gamma_2_next  = min(max(Gamma_2_next , Gamma_2_Min(idx)), Gamma_2_Max(idx));\nend\n\n\n%% ----------------------dihat_Updata----------------------\n\nd1hat_dot = diag(gamma_d1) * e2;\nd2hat_dot = diag(gamma_d2) * e3;\nd1hat_next = d1hat_dot * ts + d1hat(:);\nd2hat_next = d2hat_dot * ts + d2hat(:);\nd1max = ones(3 ,1) * 1e2;\nd2max = ones(3 ,1) * 5e-4;\nd1min = -d1max;\nd2min = -d2max;\nfor idx = 1 : 3\n   if d1hat_next(idx) > d1max(idx)\n       d1hat_next(idx) = d1max(idx);\n   end\n    if d1hat_next(idx) < d1min(idx)\n       d1hat_next(idx) = d1min(idx);\n   end\n\n   if d2hat_next(idx) > d2max(idx)\n       d2hat_next(idx) = d2max(idx);\n    end\n    if d2hat_next(idx) < d2min(idx)\n       d2hat_next(idx) = d2min(idx);\n    end\nend\nif sw_d1hat == 0\n    d1hat_next = zeros(3,1);\nend\nif sw_d2hat == 0\n    d2hat_next = zeros(3,1);\nend\n\n%%\n% Q to U\nPr = 0;                                     \nkq1 = 1.069e-9;                         \t\nkq2 = 1.069e-9;                           \t\nk = 10;                                    \t\n\nif QLd > 0 % forword\n    Delta_p1 = Ps - Pi;\n    Delta_p2 = Po - Pr;\nelse % backspacings\n    Delta_p1 = Pi - Pr;\n    Delta_p2 = Ps - Po;\nend\n\nXv = QLd ./ (Ai./Vi.*kq1.*sqrt(Delta_p1) + Ao./Vo.*kq2.*sqrt(Delta_p2));\nU = 1./k .* Xv;          \n\nUmax = 5;\nfor idx = 1 : 3\n    if U(idx) > Umax\n        U(idx) = Umax;\n    end\n    if U(idx) < -Umax\n        U(idx) = -Umax;\n    end\nend\n\n\n\n\n%%  ————————detect——————————\n% F组：每行是一个动作的数据列\nF_Swing = [FLd(1); FLda1(1); FLds1(1); FLda2(1)];\nF_Boom  = [FLd(2); FLda1(2); FLds1(2); FLda2(2)];\nF_Stick = [FLd(3); FLda1(3); FLds1(3); FLda2(3)];\n\n% Q组\nQ_Swing = [QLd(1); QLda1(1); QLds1(1); QLda2(1)];\nQ_Boom  = [QLd(2); QLda1(2); QLds1(2); QLda2(2)];\nQ_Stick = [QLd(3); QLda1(3); QLds1(3); QLda2(3)];\n\ntau = J_h * FL;" ("Base Controller")("q1"=w372, "q2"=w334, "q3"=w333, "alpha1"=w370, "alpha2"=w369, "alpha3"=w366, "pi1"=w364, "pi2"=w355, "pi3"=w356, "po1"=w357, "po2"=w358, "po3"=w359, "ts"=w346, "Ps"=w354, "Desired_Swing"=w337, "Desired_Boom"=w336, "Desired_Stick"=w335, "K1"="K1", "K2"="K2", "K3"=w322, "q_dot_f"=w276, "q_f"=w277, "Desired_q_Swing"=w330, "Desired_q_Boom"=w331, "Desired_q_Stick"=w332, "sw_QLda1"="sw_QLda1", "sw_FLda1"="sw_FLda1", "Theta_s1_init"="Theta_s1_init", "Theta_s2_init"=w315, "gamma_d1"="gamma_d1", "gamma_d2"=w325, "d1hat"=w321, "d2hat"=w319, "sw_d1hat"="sw_d1hat", "sw_d2hat"="sw_d2hat", "X1_f"=w314, "X2_f"=w313, "Gamma_1"=w264, "Theta_Stick_F_hat"=w308, "Gamma_2"=w262, "Theta_Stick_Q_hat"=w306, "Gamma_1_Swing"=w272, "Gamma_1_Boom"=w268, "Gamma_2_Swing"=w270, "Gamma_2_Boom"=w266, "Theta_Swing_F_hat"=w304, "Theta_Swing_Q_hat"=w302, "Theta_Boom_Q_hat"=w299, "Theta_Boom_F_hat"=w300, "w1"="w1", "w2"="w2", "sw_Y_Q"="sw_Y_Q", "Stop_Theta_Update"="Stop\nTheta_Update", "Use_Preset_Theta"="Use\nPreset_Theta") -> ("q_dot_f_next"=w273:dbl[], "q_f_next"=w274:dbl[], "U"=w342:dbl[], "d1hat_next"=w320:dbl[], "d2hat_next"=w318:dbl[], "X2_f_next"=w312:dbl[], "X1_f_next"=w311:dbl[], "Gamma_1_next"=w263:dbl, "Theta_Stick_F_hat_next"=w252:dbl[], "Theta_Stick_Q_hat_next"=w249:dbl[], "Gamma_2_next"=w261:dbl, "Gamma_1_Swing_next"=w271:dbl, "Gamma_2_Swing_next"=w269:dbl, "Gamma_1_Boom_next"=w267:dbl, "Gamma_2_Boom_next"=w265:dbl, "Theta_Swing_F_hat_next"=w303:dbl[], "Theta_Swing_Q_hat_next"=w301:dbl[], "Theta_Boom_Q_hat_next"=w245:dbl[], "Theta_Boom_F_hat_next"=w246:dbl[], "Epsilon_1"=w295:cdb[], "Epsilon_2"=w293:cdb[], "e2"=→"e2":dbl[], "e3"=→"e3":dbl[], "tau"=w231:dbl[], "F_Swing"=w292:cdb[], "F_Boom"=w283:cdb[], "F_Stick"=w282:cdb[], "Q_Swing"=w284:cdb[], "Q_Stick"=w286:cdb[], "Q_Boom"=w285:cdb[], "e2_e3"=→"e2_e3":dbl[])  [unwired: 1 in, 1 out]
    "ARC_U" <- w342
    "Theta_Stick_F_hat_next" <- w252
    "Theta_Stick_Q_hat_next" <- w249
    "Theta_Swing_F_hat_next" <- w303
    "Theta_Swing_Q_hat_next" <- w301
    "Theta_Boom_F_hat_next" <- w246
    "Theta_Boom_Q_hat_next" <- w245
    n202 = Array To Cluster ("数组至簇转换")(array=w286) -> (cluster=→"Q_Stick":T11)
    n203 = Array To Cluster ("数组至簇转换")(array=w285) -> (cluster=→"Q_Boom":T12)
    n204 = Array To Cluster ("数组至簇转换")(array=w284) -> (cluster=→"Q_Swing":T13)
    n205 = Array To Cluster ("数组至簇转换")(array=w282) -> (cluster=→"F_Stick":T14)
    n206 = Array To Cluster ("数组至簇转换")(array=w283) -> (cluster=→"F_Boom":T15)
    n207 = Array To Cluster ("数组至簇转换")(array=w292) -> (cluster=→"F_Swing":T16)
    n208 = feedback-in #4(w274) -> ()
    n209 = feedback-in #5(w273) -> ()
    n210 = feedback-in #6(w246) -> ()
    n211 = feedback-in #7(w245) -> ()
    n212 = feedback-in #8(w301) -> ()
    n213 = feedback-in #9(w249) -> ()
    n214 = feedback-in #10(w271) -> ()
    n215 = feedback-in #11(w269) -> ()
    n216 = feedback-in #12(w267) -> ()
    n217 = feedback-in #13(w265) -> ()
    n218 = feedback-in #14(w263) -> ()
    n219 = feedback-in #15(w261) -> ()
    n220 = feedback-in #16(w303) -> ()
    n221 = feedback-in #17(w252) -> ()
    n222 = shared-variable ".\\sharedV.lvlib\\Actual_tau"(w231) -> ()  [unwired: 1 in, 1 out]
    n223 = feedback-in #18(w320) -> ()
    n224 = feedback-in #19(w318) -> ()
    n225 = feedback-in #20(w311) -> ()
    n226 = feedback-in #21(w312) -> ()
    n227 = Array Size ("数组大小")(array=w342) -> ()  [unwired: 1 out]
    n228 = Index Array ("索引数组")(array=w342, index=1) -> (element=w338:dbl)
    n229 = Index Array ("索引数组")(array=w342, index=0) -> (element=w343:dbl)
    n230 = Index Array ("索引数组")(array=w342, index=2) -> (element=w339:dbl)
    n231 = shared-variable ".\\sharedV.lvlib\\ARC_U_Swing"(w343) -> ()  [unwired: 1 in, 1 out]
    n232 = Array To Cluster ("数组至簇转换")(array=w295) -> (cluster=→"Esti_e1":T17)
    n233 = Array To Cluster ("数组至簇转换")(array=w293) -> (cluster=→"Esti_e2":T18)
    n234 = expression code="(x/pi)*180.0" ("弧度转换至角度")(w274) -> (w229:dbl[])
    n235 = expression code="(x/pi)*180.0" ("弧度转换至角度")(w273) -> (w230:dbl[])
    n236 = shared-variable ".\\sharedV.lvlib\\ARC_U_Boom"(w338) -> ()  [unwired: 1 in, 1 out]
    n237 = shared-variable ".\\sharedV.lvlib\\ARC_U_Stick"(w339) -> ()  [unwired: 1 in, 1 out]
    n238 = shared-variable ".\\sharedV.lvlib\\q_dot_f"(w230) -> ()  [unwired: 1 in, 1 out]
    n239 = shared-variable ".\\sharedV.lvlib\\q_f"(w229) -> ()  [unwired: 1 in, 1 out]
    n240 = Array To Cluster ("数组至簇转换")(array=w249) -> (cluster=→"Theta_Stick_Q_hat_next":T19)
    n241 = Array To Cluster ("数组至簇转换")(array=w252) -> (cluster=→"Theta_Stick_F_hat_next":T1)
    n242 = Array To Cluster ("数组至簇转换")(array=w245) -> (cluster=→"Theta_Boom_Q_hat_next":T20)
    n243 = Array To Cluster ("数组至簇转换")(array=w246) -> (cluster=→"Theta_Boom_F_hat_next":T21)
    n244 = node-c288() -> ()  [unwired: 1 in, 1 out]
  }
  n245 = node-c288(w8) -> ()  [unwired: 1 out]
